vi "RunTest_NO.vi"(8 "error in (no error)":errorcluster, 11 "Prueba04 in":refnum<class "Prueba04.lvclass">) -> (0 "error out":errorcluster, 2 "resultado":string, 3 "Prueba04 out":refnum<class "Prueba04.lvclass">)   [LabVIEW 2019, in "Prueba04.lvclass"]
uses:
  Prueba04.lvclass
  Prueba/Prueba.lvclass
  Prueba/Queues/Private Controls/Estados.ctl
  Prueba/Queues/Private Controls/Control HMI Data Cluster.ctl
  Prueba/Queues/Private Controls/Queue FGV Action.ctl
  Prueba/Controles/FrecAmpGEN.ctl
  Control/Slide.ctl
panel:
  out "fila actual Z":i32
  out "frec_generar_Z2":string
  out "volt_generar_Z2":string
  out "frec_ref_Z_2":string="inicio"
  out "Vref_Z":dbl
  out "IndicadorAjuste_Z":dbl caption="Ajuste de amplitud [mV]"
  out "frecZ1":dbl
  out "cumple_no_cumple_Z":bool
  out "cumple_no_cumple_C":bool
  out "fila actual C":i32
  out "frec_generar_C2":string
  out "volt_generar_C2":string
  out "frec_ref_C":string="inicio"
  out "frecC1":dbl
  out "IndicadorAjuste_C":dbl caption="Ajuste de amplitud [mV]"
  out "Vref_C":dbl
  out "cumple_no_cumple_A":bool
  out "error out 2":errorcluster
  out "ponderacion_Z":bool
  out "ponderacion_C":bool
  out "volt_generar_A2":string
  out "FrecAmpGEN":T1
  out "Vref_A 2":dbl
  out "frecA1":dbl
  out "frec_generar_C2":string
  out "Voltajes_Ref_Z":string[](array[string])
  out "Voltajes_Ref_C":string[](array[string])
  out "fila actual Z":i32
  out "fila actual C":i32
  out "frec_ref_Z":string="inicio"
  out "frec_ref_C":string="inicio"
  out "frec_generar_A2":string
  out "fila actual A":i32
  out "Voltajes_Ref_A":string[](array[string])
  out "frec_ref_A":string="inicio"
  out "Vref_A":dbl
  out "IndicadorAjuste_A":dbl caption="Ajuste de amplitud [mV]"
  out "ponderacion_A":bool
  out "Tab":T2(tab)
  in  "go_A":bool
  in  "go_C":bool
  in  "go_Z":bool
  in  "seguir":bool
  out "no_cumple_prueba04":bool
  out "cumple_prueba04":bool
  out "estado_ensayo_A":string="Ensayo ya realizado"
  out "estado_ensayo_C":string="Ensayo ya realizado"
  out "estado_ensayo_Z":string="Ensayo ya realizado"
  in  "cb_frec_A_1":string(combo)="1000"
  in  "guardar_Vref_A":bool
  out "niveldBA_1":dbl=95.0
  out "rangoRefA_1":dbl=140.0
  in  "generarA1":bool
  in  "VoltAjuste_A":T3 caption="Ajuste de amplitud [mV]" scale=0.0..10.0
  out "voltMonA_1":dbl format="%#.1f"
  out "frecMonA_1":dbl format="%#.1f"
  in  "ir a resultados_A":bool
  in  "cb_frec_A_2":string(combo)="31,5"
  out "voltaje_A":dbl
  in  "generarA2":bool
  out "cumple_A":bool
  out "no_cumple_A":bool
  in  "ir a inicio desde A":bool
  in  "Tabla_A":string[][](table)
  out "voltMonA_2":dbl format="%#.1f"
  out "frecMonA_2":dbl format="%#.1f"
  in  "cb_frec_C_1":string(combo)="1000"
  in  "guardar_Vref_C":bool
  out "niveldBC_1":dbl
  out "rangoRefC_1":dbl
  in  "generarC1":bool
  in  "VoltAjuste_C":T3 caption="Ajuste de amplitud [mV]" scale=0.0..10.0
  out "voltMonC_1":dbl
  out "frecMonC_1":dbl
  in  "ir a resultados_C":bool
  in  "cb_frec_C_2":string(combo)="31,5"
  out "voltaje_C":dbl
  in  "generarC2":bool
  out "voltMonC_2":dbl
  out "frecMonC_2":dbl
  in  "Tabla_C":string[][](table)
  in  "ir a inicio desde C":bool
  out "cumple_C":bool
  out "no_cumple_C":bool
  in  "cb_frec_Z_1":string(combo)="1000"
  out "niveldBZ_1":dbl
  out "rangoRefZ_1":dbl
  in  "generarZ1":bool
  in  "VoltAjuste_Z":T3 caption="Ajuste de amplitud [mV]" scale=0.0..10.0
  out "voltMonZ_1":dbl
  out "frecMonZ_1":dbl
  in  "ir a resultados _Z":bool
  in  "guardar_Vref_Z":bool
  in  "cb_frec_Z_2":string(combo)="31,5"
  out "voltaje_Z":dbl
  in  "generarZ2":bool
  in  "ir a inicio desde Z":bool
  in  "Tabla_Z":string[][](table)
  out "voltMonZ_2":dbl
  out "frecMonZ_2":dbl
  out "cumple_Z":bool
  out "no_cumple_Z":bool
  # "Cumple"
  # "No Cumple"
  # "Ensayo Eléctrico Ponderación A"
  # "Ensayo Eléctrico Ponderación B"
  # "Ensayo Eléctrico Ponderación Z"
  # "Ensayo Eléctrico Ponderación A – Selección de Señal de referencia"
  # "Elección Señal de Referencia\nsegún marca y modelo de sonómetro"
  # "Nivel en dB"
  # "Rango Referencia"
  # "Frecuencia"
  # "Monitoreo"
  # "Frecuencia"
  # "Hz"
  # "Voltaje"
  # "V"
  # "Ensayo Eléctrico Ponderación A – Tabla de Resultados"
  # "Cumple"
  # "No Cumple"
  # "Hz"
  # "mV"
  # "Voltaje"
  # "Frecuencia"
  # "Ponderación A"
  # "Monitoreo"
  # "Frecuencia"
  # "Hz"
  # "Voltaje"
  # "V"
  # "Ensayo Eléctrico Ponderación C – Selección de Señal de referencia"
  # "Elección Señal de Referencia\nsegún marca y modelo de sonómetro"
  # "Nivel en dB"
  # "Rango Referencia"
  # "Frecuencia"
  # "Monitoreo"
  # "Frecuencia"
  # "Hz"
  # "Voltaje"
  # "V"
  # "Ensayo Eléctrico Ponderación C – Tabla de Resultados"
  # "Cumple"
  # "No Cumple"
  # "Hz"
  # "mV"
  # "Voltaje"
  # "Frecuencia"
  # "Monitoreo"
  # "Frecuencia"
  # "Hz"
  # "Voltaje"
  # "V"
  # "Ponderación C"
  # "Ensayo Eléctrico Ponderación Z – Selección de Señal de referencia"
  # "Elección Señal de Referencia\nsegún marca y modelo de sonómetro"
  # "Nivel en dB"
  # "Rango Referencia"
  # "Frecuencia"
  # "Monitoreo"
  # "Frecuencia"
  # "Hz"
  # "Voltaje"
  # "V"
  # "Ensayo Eléctrico Ponderación Z – Tabla de Resultados"
  # "Cumple"
  # "No Cumple"
  # "Hz"
  # "mV"
  # "Voltaje"
  # "Frecuencia"
  # "Ponderación Z"
  # "Monitoreo"
  # "Frecuencia"
  # "Hz"
  # "Voltaje"
  # "V"
  # "4. Ensayo  de las ponderaciones frecuenciales con señales eléctricas. IEC 61672-3: 2006 Cláusula 12"
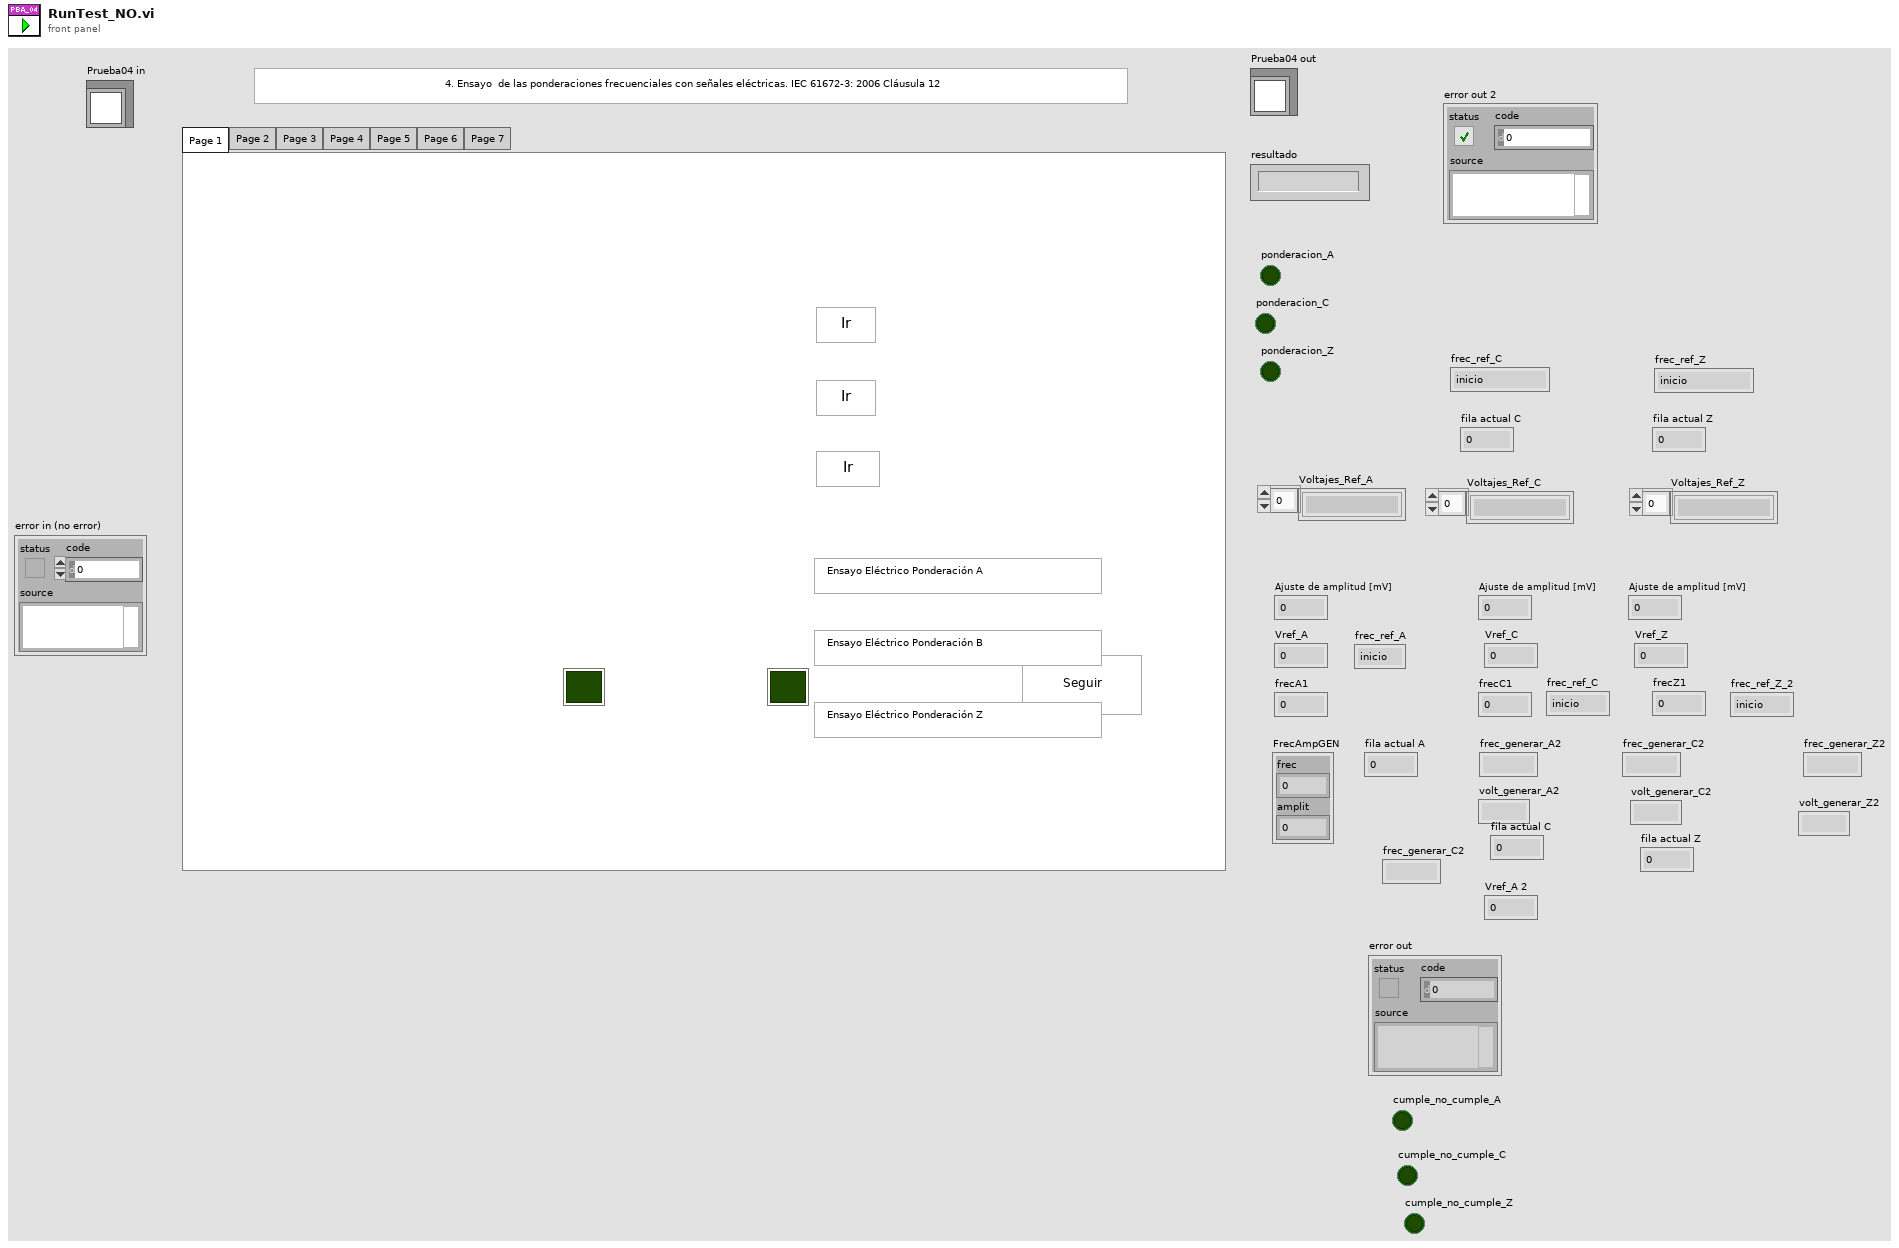
[diagram p1: front panel]
types:
  T1 = typedef "Prueba04.lvclass/FrecAmpGEN.ctl" = cluster{"frec":dbl, "amplit":dbl}
  T2 = enum32{"Page 1", "Page 2", "Page 3", "Page 4", "Page 5", "Page 6", "Page 7"}
  T3 = typedef "Prueba04.lvclass/Slide.ctl" = dbl
  T4 = cluster{"Medido":dbl, "Ref":dbl, "Incert_exp":dbl, "Tol+":dbl, "Tol-":dbl, "fila":i32}
  T5 = typedef "Queue FGV Action.ctl" = enum16{"Set", "Get", "Release"}
  T6 = enum8{"Enabled", "Disabled", "Disabled and Grayed Out"}
  T7 = typedef "Control HMI Data Cluster.ctl" = cluster{"Estados":T8, "Data":variant}
  T8 = typedef "Estados.ctl" = enum16{"CargaReferencias", "LeerArchivoConfiguracion", "RevisaTipoGenerador", "inicio", "conf_instru", "escribe_frec", "lee_BD", "lee_referencia", "guardarVrefA", "guardarVrefC", "guardarVrefZ", "FrecAmp_A1", "FrecAmp_C1", "FrecAmp_Z1", "FrecAmp_A2", "FrecAmp_C2", "FrecAmp_Z2", "iniciarGEN", "monitoreo", "detenerGEN", "crea_voltajes_prueba_A", "crea_voltajes_prueba_C", "crea_voltajes_prueba_Z", "voltajeInicialA2", "voltajeInicialC2", "voltajeInicialZ2", "actualizarVrefA", "actualizarVrefC", "actualizarVrefZ", "ingresaMedicionesA", "ingresaMedicionesC", "ingresaMedicionesZ", "cumplimiento", "listo_evaluar", "evaluar", "final", "guardaMedicionesA", "guardaMedicionesC", "guardaMedicionesZ", "ultimaFrec", "generaA2", "detieneA2", "salir", "Error"}
  T9 = cluster{"Medido":dbl, "Error":dbl, "Ref":dbl, "Incert_exp":dbl, "Tol+":dbl, "Tol-":dbl, "fila":i32}
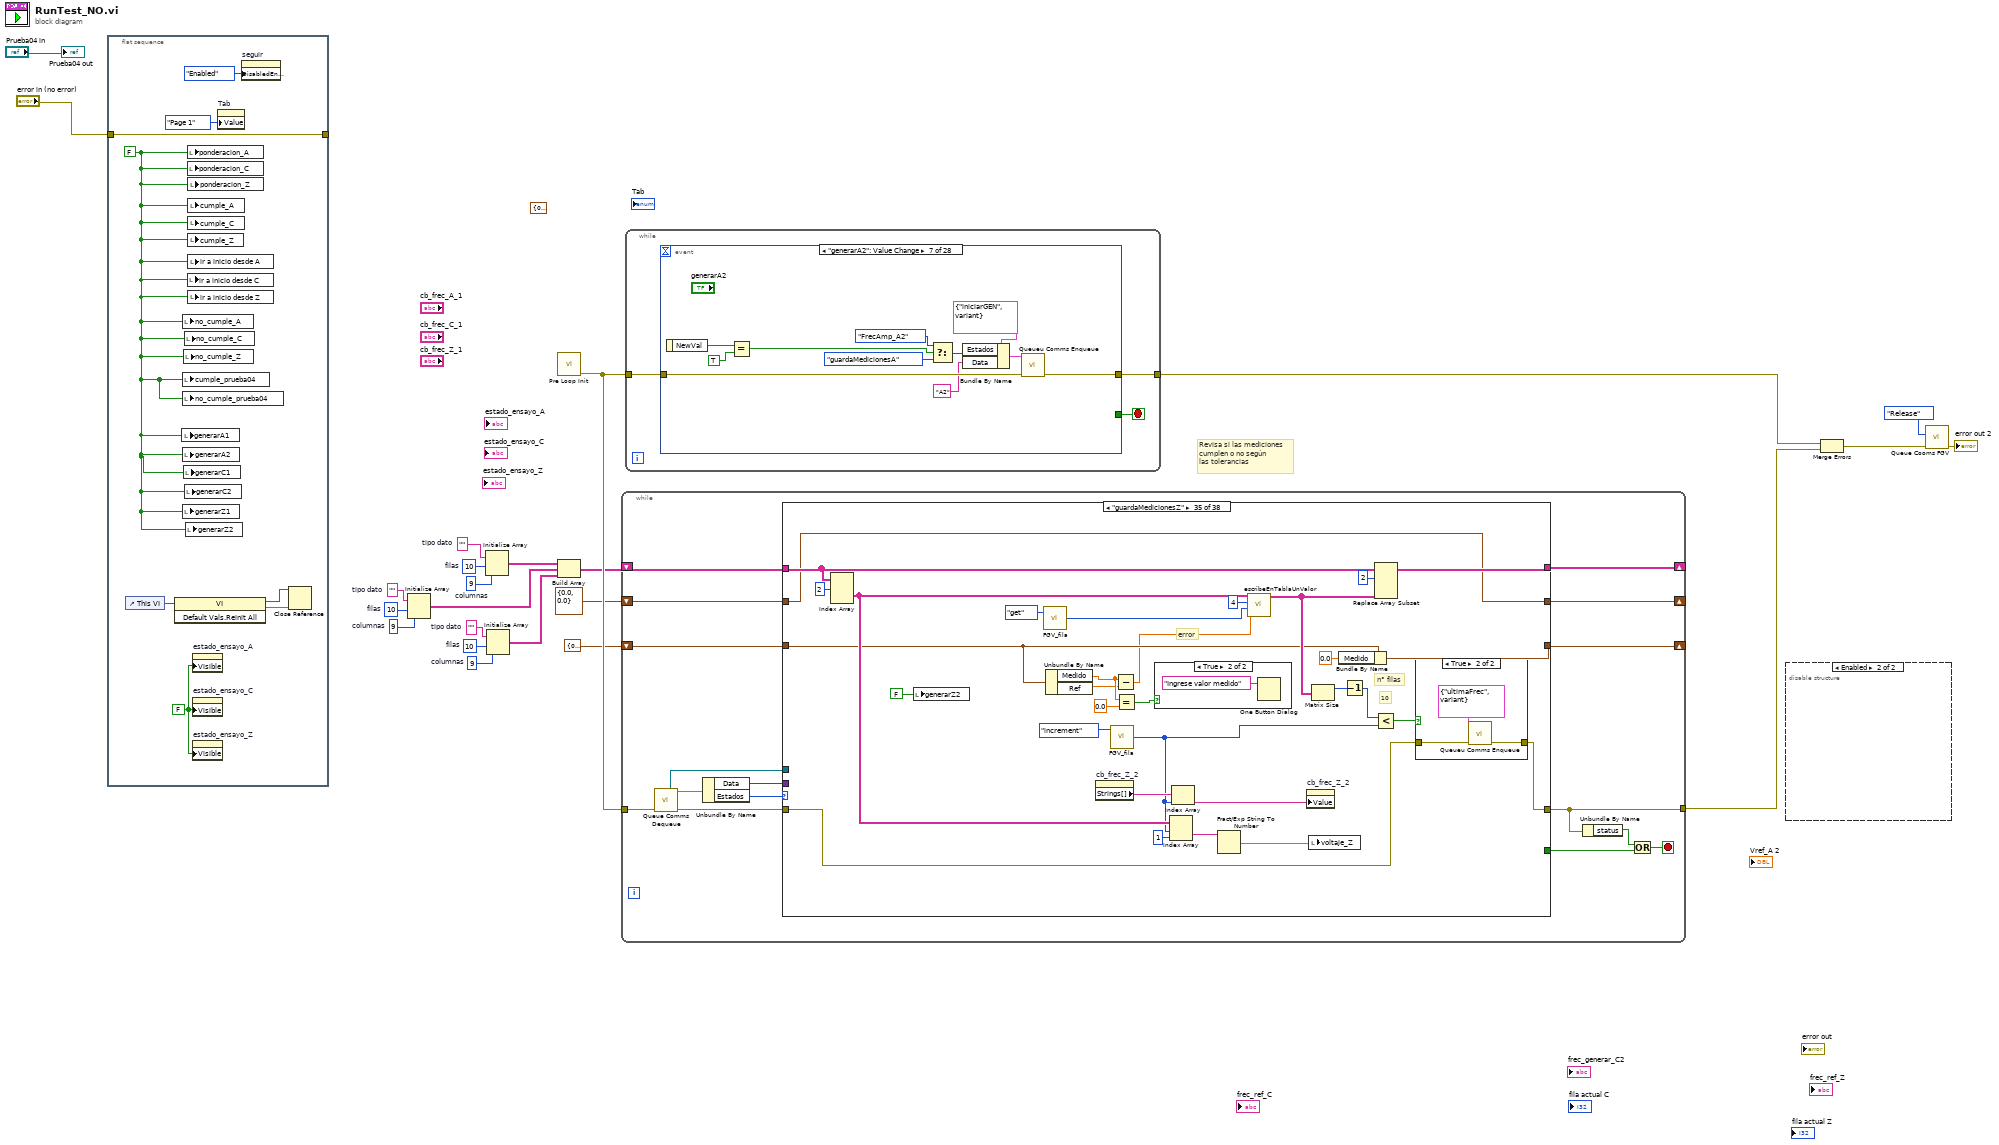
[diagram p0: block diagram]
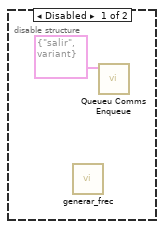
[diagram p2: hidden frame]
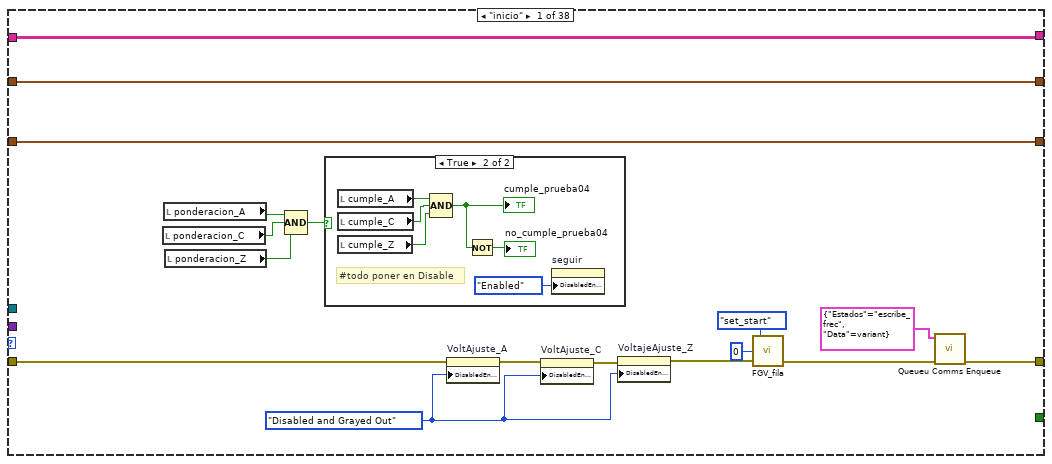
[diagram p3: hidden frame]
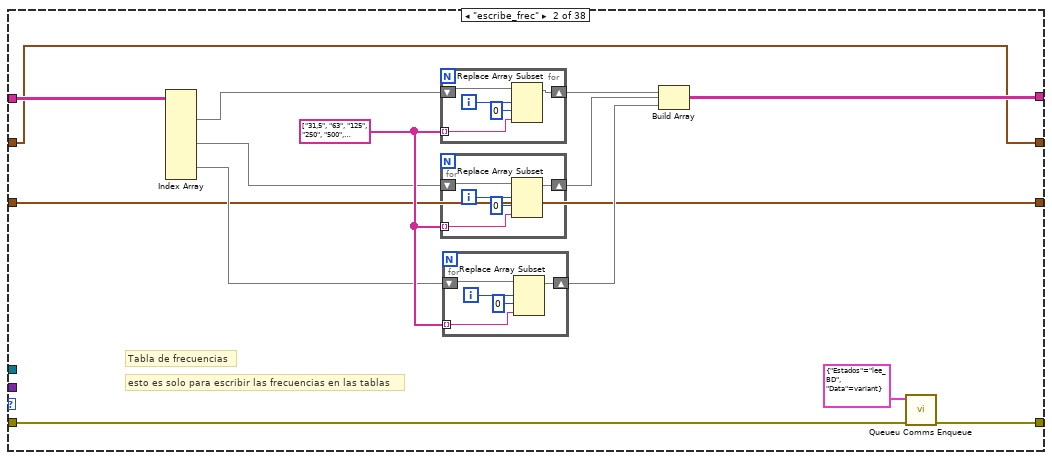
[diagram p5: hidden frame]
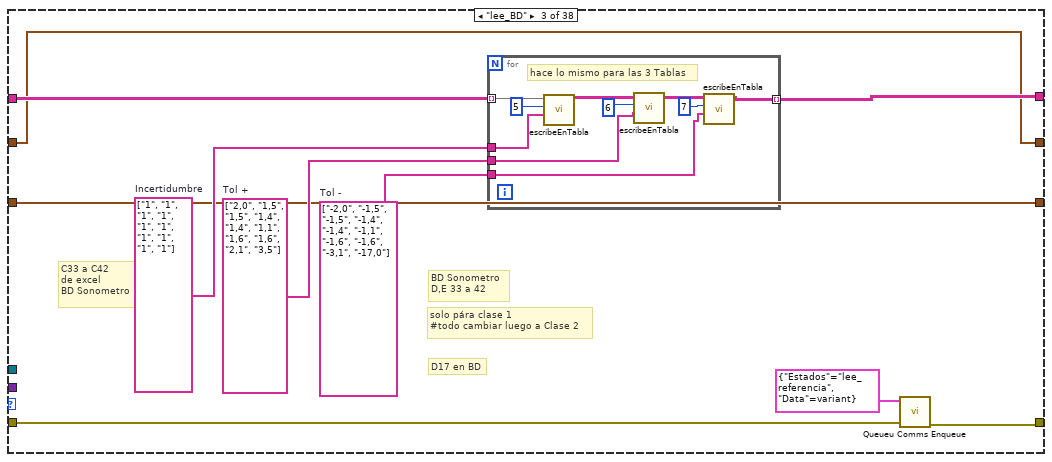
[diagram p6: hidden frame]
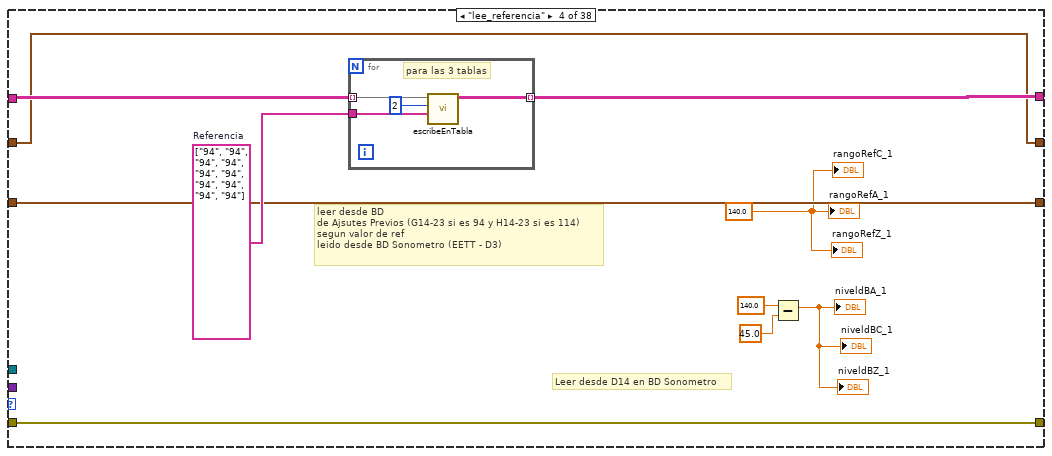
[diagram p7: hidden frame]
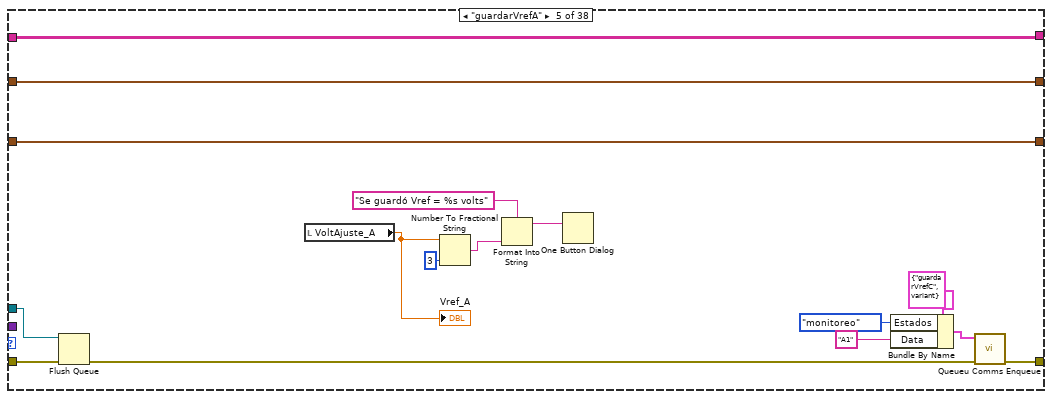
[diagram p8: hidden frame]
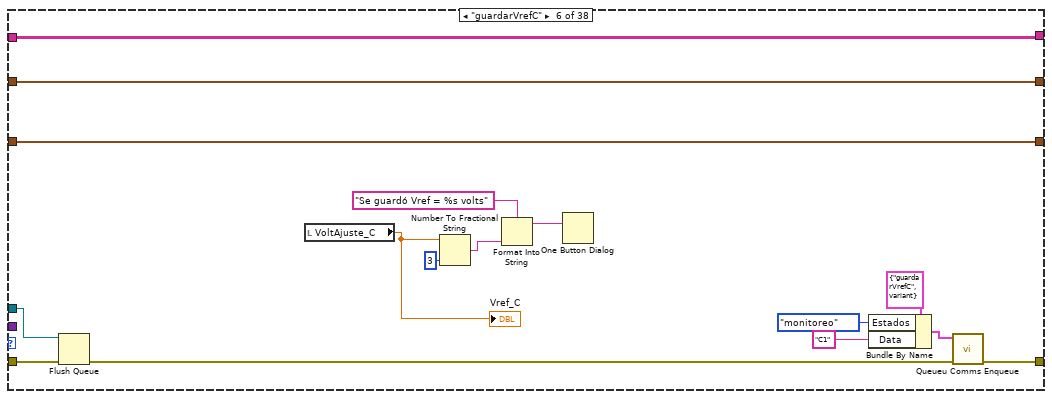
[diagram p9: hidden frame]
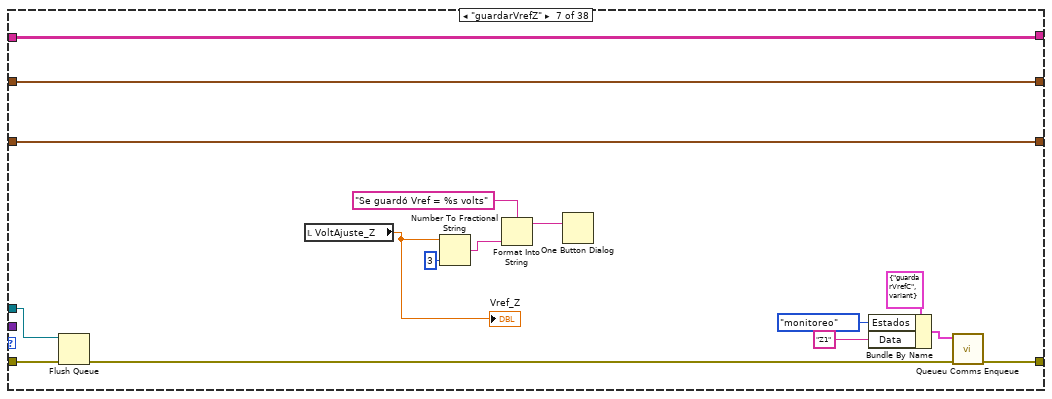
[diagram p10: hidden frame]
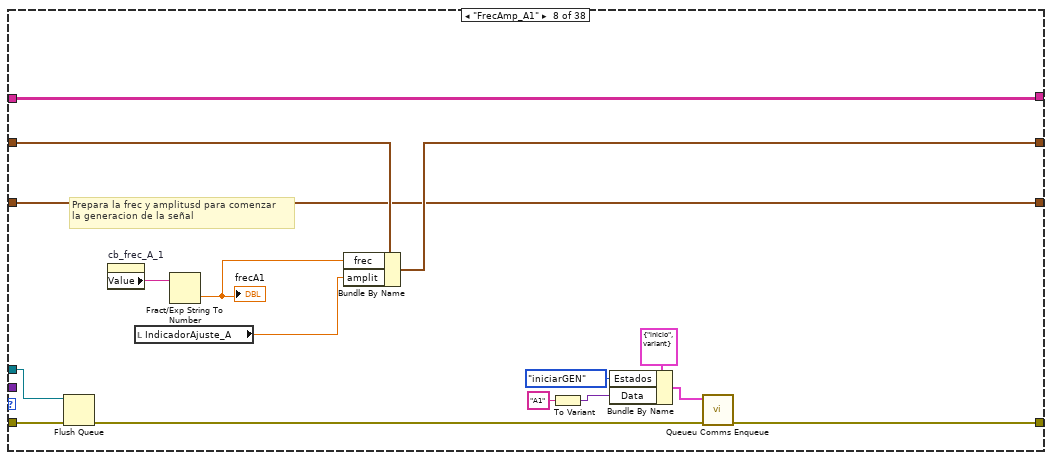
[diagram p11: hidden frame]
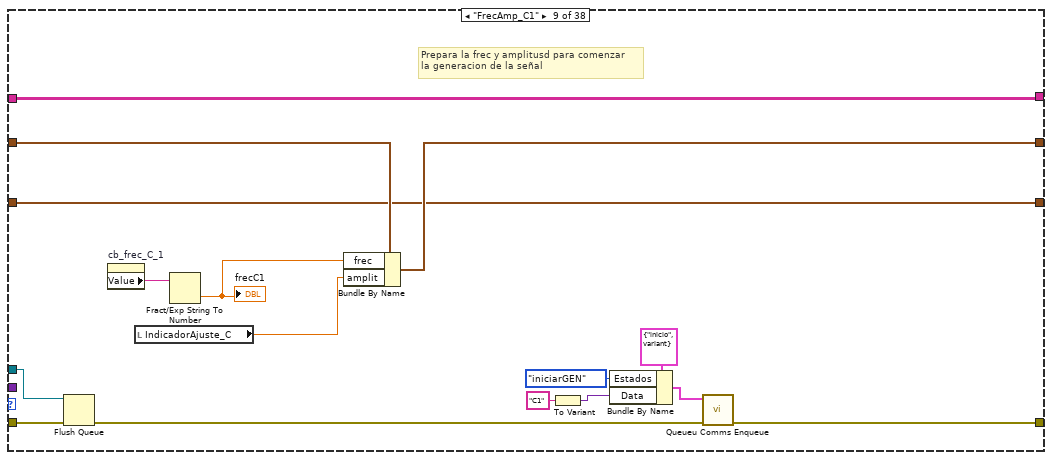
[diagram p12: hidden frame]
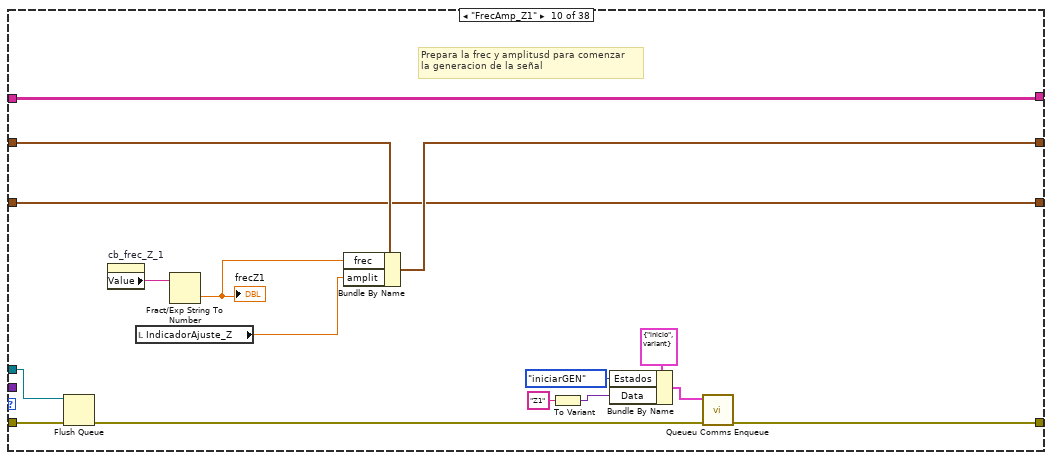
[diagram p13: hidden frame]
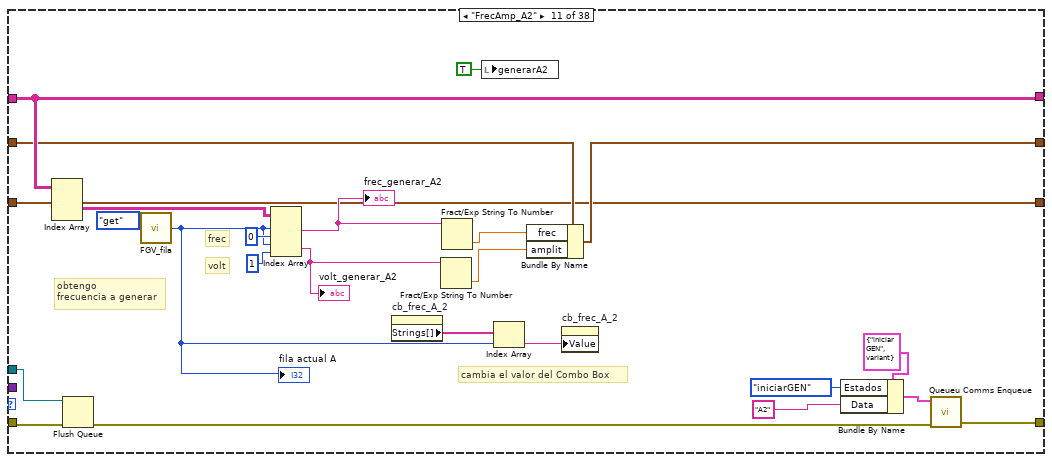
[diagram p14: hidden frame]
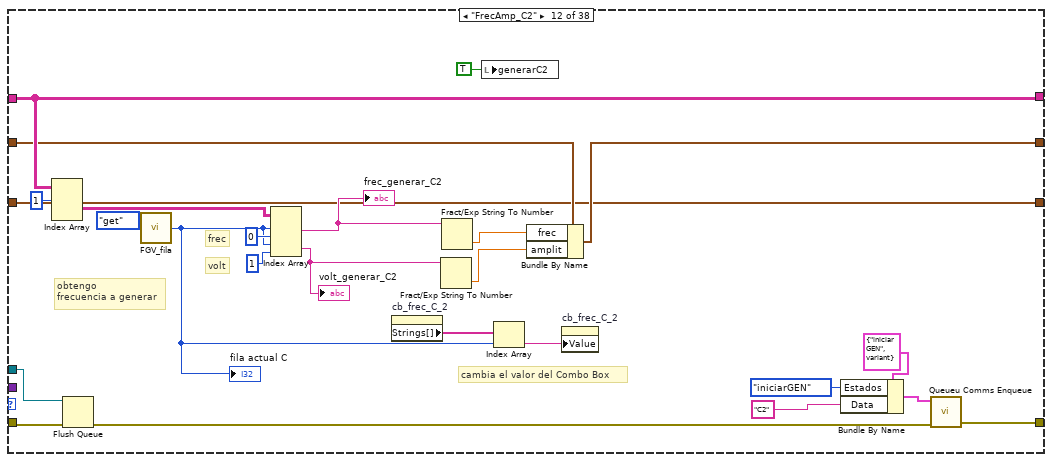
[diagram p15: hidden frame]
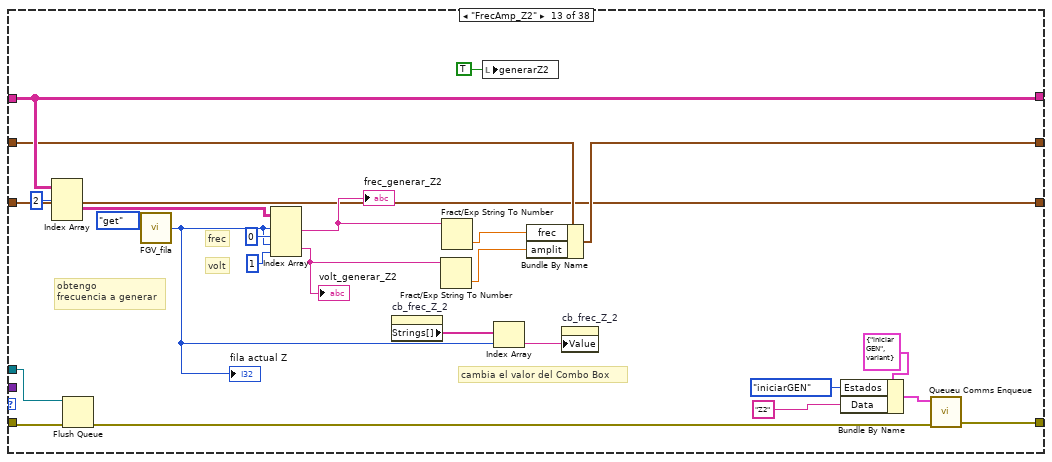
[diagram p16: hidden frame]
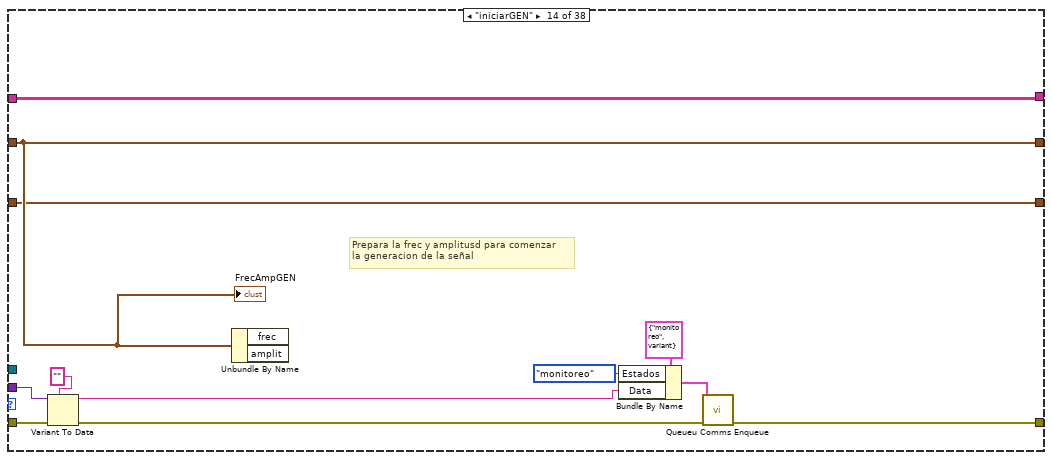
[diagram p17: hidden frame]
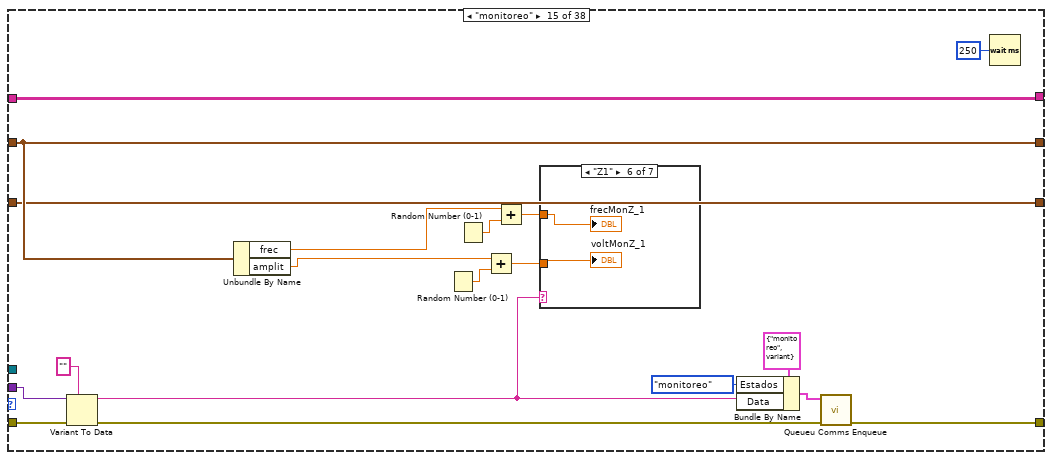
[diagram p18: hidden frame]
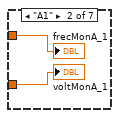
[diagram p20: hidden frame]
diagram:
  w12 = 9  # columnas
  w13 = 10  # filas
  w11 = ""  # tipo dato
  w9 = 9  # columnas
  w8 = 10  # filas
  w10 = ""  # tipo dato
  w6 = 9  # columnas
  w7 = 10  # filas
  w5 = ""  # tipo dato
  (unwired) T4 {"Medido"=0.0, "Ref"=0.0, "Incert_exp"=0.0, "Tol+"=0.0, "Tol-"=0.0, "fila"=0}
  # "Revisa si las mediciones\ncumplen o no según\nlas tolerancias"
  n1 = flat-sequence {
    tunnel: "error in (no error)" -> [w30]
    tunnel: [w30] -> _
    frame #0 {
      w24 = FALSE ("Visible")
      w25 = FALSE ("cumple_A")
      n2 = control-ref of="This VI"() -> (w27:refnum<vi>)
      n3 = invoke class="VI" method="Default Vals.Reinit All"(reference=w27) -> (reference out=w26:refnum<vi>, error out=w28:errorcluster)  [unwired: 2 in, 1 out]
      n4 = local write "generarA1"(w25) -> ()
      n5 = local write "no_cumple_A"(w25) -> ()
      n6 = local write "cumple_prueba04"(w25) -> ()
      n7 = local write "no_cumple_prueba04"(w25) -> ()
      n8 = local write "generarA2"(w25) -> ()
      n9 = local write "generarZ1"(w25) -> ()
      n10 = local write "no_cumple_Z"(w25) -> ()
      n11 = local write "generarC1"(w25) -> ()
      n12 = local write "no_cumple_C"(w25) -> ()
      n13 = local write "generarC2"(w25) -> ()
      n14 = local write "generarZ2"(w25) -> ()
      n15 = local write "ponderacion_A"(w25) -> ()
      n16 = local write "ponderacion_C"(w25) -> ()
      n17 = local write "ir a inicio desde C"(w25) -> ()
      n18 = local write "ponderacion_Z"(w25) -> ()
      n19 = local write "cumple_A"(w25) -> ()
      n20 = local write "cumple_C"(w25) -> ()
      n21 = local write "cumple_Z"(w25) -> ()
      n22 = local write "ir a inicio desde A"(w25) -> ()
      n23 = local write "ir a inicio desde Z"(w25) -> ()
      n24 = property on="estado_ensayo_A" class="Str"("Visible"=w24) -> ()  [unwired: 2 in, 2 out]
      n25 = property on="estado_ensayo_C" class="Str"("Visible"=w24) -> ()  [unwired: 2 in, 2 out]
      n26 = property on="estado_ensayo_Z" class="Str"("Visible"=w24) -> ()  [unwired: 2 in, 2 out]
      n27 = property on="Tab" class="TabCtl (strict)"("Value"=T2."Page 1" ("Tab_Prueba04")) -> ()  [unwired: 2 in, 2 out]
      n28 = property on="seguir" class="Bool"("DisabledEnum"=T6."Enabled" ("Disabled")) -> ()  [unwired: 2 in, 2 out]
      n29 = Close Reference(reference=w26, error in (no error)=w28) -> ()  [unwired: 1 out]
    }
  }
  n30 = Initialize Array(w10, w8, w9) -> (w15:string[][])
  n31 = Initialize Array(w5, w7, w6) -> (w14:string[][])
  n32 = Initialize Array(w11, w13, w12) -> (w16:string[][])
  n33 = call "Pre Loop Init.vi"() -> ("error out"=w21:errorcluster)  [unwired: 11 in]
  n34 = Build Array(w14, w15, w16) -> (w4:string[][][])
  n35 = while {
    tunnel: w21 -> [w45]
    tunnel: [w43] -> w19
    shift-right: [w38] -> _
    shift-left: w4 -> [w39]
    shift-right: [w36] -> _
    shift-left: T1 {"frec"=0.0, "amplit"=0.0} ("ParamGeneracion") -> [w37]
    shift-right: [w32] -> _
    shift-left: T4 {"Medido"=0.0, "Ref"=0.0, "Incert_exp"=0.0, "Tol+"=0.0, "Tol-"=0.0, "fila"=0} -> [w33]
    stop <- w40 stop-if-true
    n36 = call "Queue Comms Dequeue.vi"("error in"=w45) -> ("error out"=w44:errorcluster, "Data Out"=w35:T7, "queue out"=w34:refnum<queue>)  [unwired: 8 in]
    n37 = Unbundle By Name(w35) -> ("Data"=w46:variant, "Estados"=w47:T8)
    n38 = case shown="\"guardaMedicionesZ\"" w47 {
      tunnel: w46 -> [_ _ _ _ _ _ _ _ _ _ _ _ _ w306 w324 _ _ _ _ _ _ _ _ _ _ w515 w538 w561 w578 w594 w656 _ _ _ _ _ _ _]
      tunnel: [_ _ _ _ _ _ _ _ _ _ _ _ _ _ _ _ _ _ _ _ _ _ _ _ _ _ _ _ _ _ _ _ _ _ _ _ TRUE _] -> w41
      tunnel: [w60 w74 w103 w124 w135 w155 w171 w194 w210 w226 w235 w260 w285 w313 w317 w349 w360 w387 w413 w435 w445 w451 w465 w476 w487 w510 w533 w556 w568 w596 w660 w704 w711 w749 w787 w824 w832 w837] -> w43
      tunnel: w44 -> [w49 w73 w102 w124 w144 w160 w176 w195 w211 w227 w233 w258 w283 w314 w333 w353 w361 w388 w414 w435 w445 w452 w466 w477 w488 w496 w519 w542 w579 w600 w664 w704 w712 w750 w788 w820 w832 w837]
      tunnel: w39 -> [w58 w77 w106 w126 w149 w165 w181 w197 w213 w229 w249 w274 w299 w315 w334 w354 w367 w393 w419 w441 w450 w460 w471 w482 w493 w513 w536 w559 w576 w597 w661 w703 w730 w768 w806 w828 w831 w836]
      tunnel: [w58 w76 w105 w125 w149 w165 w181 w197 w213 w229 w249 w274 w299 w315 w334 w354 w366 w392 w418 w441 w450 w460 w471 w482 w493 w512 w535 w558 w572 w597 w661 w703 w729 w767 w805 w828 w831 w836] -> w38
      tunnel: w37 -> [w57 w72 w101 w123 w143 w159 w175 w193 w209 w225 w244 w269 w294 w312 w325 w352 w359 w386 w412 w434 w444 w455 w470 w481 w492 w516 w539 w562 w581 w599 w663 w702 w720 w758 w796 w827 w830 w835]
      tunnel: [w57 w72 w101 w123 w143 w159 w175 w191 w207 w223 w239 w264 w289 w312 w325 w352 w359 w386 w412 w434 w444 w455 w470 w481 w492 w516 w539 w562 w581 w599 w663 w702 w720 w758 w796 w827 w830 w835] -> w36
      tunnel: w34 -> [_ _ _ _ w141 w158 w174 w183 w199 w215 w231 w256 w281 _ _ w348 w357 w384 w410 _ _ _ _ _ _ w494 w517 w540 _ _ _ _ _ _ _ _ _ _]
      tunnel: w33 -> [w55 w71 w100 w122 w140 w157 w173 w182 w198 w214 w230 w255 w280 w304 w316 w347 w356 w383 w409 w433 w443 w454 w469 w480 w491 w501 w524 w547 w574 w598 w662 w701 w709 w747 w785 w821 w829 w834]
      tunnel: [w55 w71 w100 w122 w140 w157 w173 w182 w198 w214 w230 w255 w280 w304 w316 w347 w356 w383 w409 w433 w443 w454 w469 w480 w491 w497 w520 w543 w573 w598 w662 w701 w707 w745 w783 w821 w829 w834] -> w32
      frame "inicio" {
        w50 = T6."Disabled and Grayed Out" ("Disabled")
        n39 = local read "ponderacion_C"() -> (w56:bool)
        n40 = local read "ponderacion_A"() -> (w63:bool)
        n41 = local read "ponderacion_Z"() -> (w64:bool)
        n42 = Compound Arithmetic op=AND(w63, w56, w64) -> (w48:bool)
        n43 = case shown="True" w48 {
          frame False {
          }
          frame True {
            # "#todo poner en Disable"
            n44 = local read "cumple_A"() -> (w70:bool)
            n45 = local read "cumple_C"() -> (w66:bool)
            n46 = local read "cumple_Z"() -> (w65:bool)
            n47 = Compound Arithmetic op=AND(w70, w66, w65) -> (w67:bool)
            "cumple_prueba04" <- w67
            n48 = Not(x=w67) -> (.not. x?=→"no_cumple_prueba04":bool)
            n49 = property on="seguir" class="Bool"("DisabledEnum"=T6."Enabled" ("Disabled")) -> ()  [unwired: 2 in, 2 out]
          }
        }
        n50 = property on="VoltAjuste_A" class="Slide (strict)"(error in=w49, "DisabledEnum"=w50) -> (error out=w53:errorcluster)  [unwired: 1 in, 1 out]
        n51 = property on="VoltAjuste_C" class="Slide (strict)"(error in=w53, "DisabledEnum"=w50) -> (error out=w52:errorcluster)  [unwired: 1 in, 1 out]
        n52 = property on="VoltajeAjuste_Z" class="Slide (strict)"(error in=w52, "DisabledEnum"=w50) -> (error out=w51:errorcluster)  [unwired: 1 in, 1 out]
        n53 = call "FGV_fila.vi"("error in (no error)"=w51, "fila_inicial"=0, "action"=enum16{"increment", "set_start", "get"}."set_start") -> ("error out"=w54:errorcluster)  [unwired: 1 in, 1 out]
        n54 = call "Queueu Comms Enqueue.vi"("error in"=w54, "Element"=T7 {"Estados"=enum."escribe_frec", "Data"=variant} ("Module Dat Cluster")) -> ("error out"=w60:errorcluster)  [unwired: 8 in, 1 out]
      }
      frame "escribe_frec" {
        w84 = string[] ["31,5", "63", "125", "250", "500", "1000", "2000", "4000", "8000", "16000"]
        # "esto es solo para escribir las frecuencias en las tablas"
        # "Tabla de frecuencias"
        n55 = Index Array(array=w77) -> (element #1=w78:string[][], element #2=w79:string[][], element #3=w80:string[][])  [unwired: 9 in]
        n56 = for {
          shift-right: [w98] -> w81
          shift-left: w78 -> [w99]
          tunnel: w84 -> [w95] mode=indexing
          i -> [w97]
          n57 = Replace Array Subset(array=w99, new element=w95, index (row)=w97, index (col)=0 ("disabled index (col)")) -> (w98:string[][])
        }
        n58 = for {
          shift-right: [w93] -> w82
          shift-left: w79 -> [w94]
          tunnel: w84 -> [w90] mode=indexing
          i -> [w92]
          n59 = Replace Array Subset(array=w94, new element=w90, index (row)=w92, index (col)=0 ("disabled index (col)")) -> (w93:string[][])
        }
        n60 = for {
          shift-right: [w88] -> w83
          shift-left: w80 -> [w89]
          tunnel: w84 -> [w85] mode=indexing
          i -> [w87]
          n61 = Replace Array Subset(array=w89, new element=w85, index (row)=w87, index (col)=0 ("disabled index (col)")) -> (w88:string[][])
        }
        n62 = Build Array(w81, w82, w83) -> (w76:string[][][])
        n63 = call "Queueu Comms Enqueue.vi"("error in"=w73, "Element"=T7 {"Estados"=enum."lee_BD", "Data"=variant} ("Module Dat Cluster")) -> ("error out"=w74:errorcluster)  [unwired: 8 in, 1 out]
      }
      frame "lee_BD" {
        w109 = string[] ["-2,0", "-1,5", "-1,5", "-1,4", "-1,4", "-1,1", "-1,6", "-1,6", "-3,1", "-17,0"]  # Tol -
        w108 = string[] ["2,0", "1,5", "1,5", "1,4", "1,4", "1,1", "1,6", "1,6", "2,1", "3,5"]  # Tol +
        w107 = string[] ["1", "1", "1", "1", "1", "1", "1", "1", "1", "1"]  # Incertidumbre
        # "D17 en BD"
        # "BD Sonometro\nD,E 33 a 42"
        # "solo pára clase 1\n#todo cambiar luego a Clase 2"
        # "C33 a C42\nde excel\nBD Sonometro"
        n64 = for {
          tunnel: w106 -> [w118] mode=indexing
          tunnel: w107 -> [w116]
          tunnel: w108 -> [w113]
          tunnel: w109 -> [w110]
          tunnel: [w111] -> w105 mode=indexing
          # "hace lo mismo para las 3 Tablas"
          n65 = call "escribeEnTabla.vi"("parametros"=w116, "col"=5, "tabla in"=w118) -> ("tabla out"=w115:string[][])  [unwired: 8 in]
          n66 = call "escribeEnTabla.vi"("parametros"=w113, "col"=6, "tabla in"=w115) -> ("tabla out"=w112:string[][])  [unwired: 8 in]
          n67 = call "escribeEnTabla.vi"("parametros"=w110, "col"=7, "tabla in"=w112) -> ("tabla out"=w111:string[][])  [unwired: 8 in]
        }
        n68 = call "Queueu Comms Enqueue.vi"("error in"=w102, "Element"=T7 {"Estados"=enum."lee_referencia", "Data"=variant} ("Module Dat Cluster")) -> ("error out"=w103:errorcluster)  [unwired: 8 in, 1 out]
      }
      frame "lee_referencia" {
        w121 = 140.0 ("rangoRefA_1")
        w127 = string[] ["94", "94", "94", "94", "94", "94", "94", "94", "94", "94"]  # Referencia
        # "Leer desde D14 en BD Sonometro"
        # "leer desde BD\nde Ajsutes Previos (G14-23 si es 94 y H14-23 si es 114)  \nsegun valor de ref\nleido desde BD Sonometro (EETT - D3)"
        n69 = for {
          tunnel: w126 -> [w133] mode=indexing
          tunnel: [w132] -> w125 mode=indexing
          tunnel: w127 -> [w130]
          # "para las 3 tablas"
          n70 = call "escribeEnTabla.vi"("parametros"=w130, "col"=2, "tabla in"=w133) -> ("tabla out"=w132:string[][])  [unwired: 8 in]
        }
        n71 = Subtract(x=140.0 ("rangoRefA_1"), y=45.0) -> (x-y=→"niveldBA_1" →"niveldBC_1" →"niveldBZ_1":dbl)
        "rangoRefA_1" <- w121
        "rangoRefC_1" <- w121
        "rangoRefZ_1" <- w121
      }
      frame "guardarVrefA" {
        n72 = Flush Queue(queue=w141, error in (no error)=w144) -> (error out=w134:errorcluster)  [unwired: 2 out]
        n73 = local read "VoltAjuste_A"() -> (w142:T3)
        "Vref_A" <- w142
        n74 = Number To Fractional String(number=w142, precision (6)=i16 3) -> (F-format string=w148:string)  [unwired: 2 in]
        n75 = Format Into String(format string="Se guardó Vref = %s volts", w148) -> (resulting string=w145:string)  [unwired: 2 in, 1 out]
        n76 = One Button Dialog(message=w145) -> ()  [unwired: 1 in, 1 out]
        n77 = Bundle By Name(cluster=T7 {"Estados"=enum."guardarVrefC", "Data"=variant} ("Module Dat Cluster"), "Estados"=Estados."monitoreo", "Data"="A1" ("format string")) -> (w139:T7)
        n78 = call "Queueu Comms Enqueue.vi"("error in"=w134, "Element"=w139) -> ("error out"=w135:errorcluster)  [unwired: 8 in, 1 out]
      }
      frame "guardarVrefC" {
        n79 = Flush Queue(queue=w158, error in (no error)=w160) -> (error out=w154:errorcluster)  [unwired: 2 out]
        n80 = local read "VoltAjuste_C"() -> (w156:T3)
        "Vref_C" <- w156
        n81 = Number To Fractional String(number=w156, precision (6)=i16 3) -> (F-format string=w164:string)  [unwired: 2 in]
        n82 = Format Into String(format string="Se guardó Vref = %s volts", w164) -> (resulting string=w161:string)  [unwired: 2 in, 1 out]
        n83 = One Button Dialog(message=w161) -> ()  [unwired: 1 in, 1 out]
        n84 = Bundle By Name(cluster=T7 {"Estados"=enum."guardarVrefC", "Data"=variant} ("Module Dat Cluster"), "Estados"=Estados."monitoreo", "Data"="C1" ("format string")) -> (w152:T7)
        n85 = call "Queueu Comms Enqueue.vi"("error in"=w154, "Element"=w152) -> ("error out"=w155:errorcluster)  [unwired: 8 in, 1 out]
      }
      frame "guardarVrefZ" {
        n86 = Flush Queue(queue=w174, error in (no error)=w176) -> (error out=w170:errorcluster)  [unwired: 2 out]
        n87 = local read "VoltAjuste_Z"() -> (w172:T3)
        "Vref_Z" <- w172
        n88 = Number To Fractional String(number=w172, precision (6)=i16 3) -> (F-format string=w180:string)  [unwired: 2 in]
        n89 = Format Into String(format string="Se guardó Vref = %s volts", w180) -> (resulting string=w177:string)  [unwired: 2 in, 1 out]
        n90 = One Button Dialog(message=w177) -> ()  [unwired: 1 in, 1 out]
        n91 = Bundle By Name(cluster=T7 {"Estados"=enum."guardarVrefC", "Data"=variant} ("Module Dat Cluster"), "Estados"=Estados."monitoreo", "Data"="Z1" ("format string")) -> (w168:T7)
        n92 = call "Queueu Comms Enqueue.vi"("error in"=w170, "Element"=w168) -> ("error out"=w171:errorcluster)  [unwired: 8 in, 1 out]
      }
      frame "FrecAmp_A1" {
        # "Prepara la frec y amplitusd para comenzar\nla generacion de la señal"
        n93 = Flush Queue(queue=w183, error in (no error)=w195) -> (error out=w184:errorcluster)  [unwired: 2 out]
        n94 = property on="cb_frec_A_1" class="CmbBox"() -> ("Value"=w196:string)  [unwired: 2 in, 2 out]
        n95 = local read "IndicadorAjuste_A"() -> (w185:dbl)
        n96 = Fract/Exp String To Number(string=w196) -> (number=w192:dbl)  [unwired: 3 in, 1 out]
        "frecA1" <- w192
        n97 = Bundle By Name(cluster=w193, "frec"=w192, "amplit"=w185) -> (w191:T1)
        n98 = To Variant(anything="A1" ("message")) -> (Variant=w186:variant)
        n99 = Bundle By Name(cluster=T7 {"Estados"=enum."inicio", "Data"=variant} ("Element"), "Estados"=Estados."iniciarGEN", "Data"=w186) -> (w188:T7)
        n100 = call "Queueu Comms Enqueue.vi"("error in"=w184, "Element"=w188) -> ("error out"=w194:errorcluster)  [unwired: 8 in, 1 out]
      }
      frame "FrecAmp_C1" {
        # "Prepara la frec y amplitusd para comenzar\nla generacion de la señal"
        n101 = Flush Queue(queue=w199, error in (no error)=w211) -> (error out=w200:errorcluster)  [unwired: 2 out]
        n102 = property on="cb_frec_C_1" class="CmbBox"() -> ("Value"=w212:string)  [unwired: 2 in, 2 out]
        n103 = local read "IndicadorAjuste_C"() -> (w201:dbl)
        n104 = Fract/Exp String To Number(string=w212) -> (number=w208:dbl)  [unwired: 3 in, 1 out]
        "frecC1" <- w208
        n105 = Bundle By Name(cluster=w209, "frec"=w208, "amplit"=w201) -> (w207:T1)
        n106 = To Variant(anything="C1" ("message")) -> (Variant=w202:variant)
        n107 = Bundle By Name(cluster=T7 {"Estados"=enum."inicio", "Data"=variant} ("Element"), "Estados"=Estados."iniciarGEN", "Data"=w202) -> (w204:T7)
        n108 = call "Queueu Comms Enqueue.vi"("error in"=w200, "Element"=w204) -> ("error out"=w210:errorcluster)  [unwired: 8 in, 1 out]
      }
      frame "FrecAmp_Z1" {
        # "Prepara la frec y amplitusd para comenzar\nla generacion de la señal"
        n109 = Flush Queue(queue=w215, error in (no error)=w227) -> (error out=w216:errorcluster)  [unwired: 2 out]
        n110 = property on="cb_frec_Z_1" class="CmbBox"() -> ("Value"=w228:string)  [unwired: 2 in, 2 out]
        n111 = local read "IndicadorAjuste_Z"() -> (w217:dbl)
        n112 = Fract/Exp String To Number(string=w228) -> (number=w224:dbl)  [unwired: 3 in, 1 out]
        "frecZ1" <- w224
        n113 = Bundle By Name(cluster=w225, "frec"=w224, "amplit"=w217) -> (w223:T1)
        n114 = To Variant(anything="Z1" ("message")) -> (Variant=w218:variant)
        n115 = Bundle By Name(cluster=T7 {"Estados"=enum."inicio", "Data"=variant} ("Element"), "Estados"=Estados."iniciarGEN", "Data"=w218) -> (w220:T7)
        n116 = call "Queueu Comms Enqueue.vi"("error in"=w216, "Element"=w220) -> ("error out"=w226:errorcluster)  [unwired: 8 in, 1 out]
      }
      frame "FrecAmp_A2" {
        # "volt"
        # "frec"
        # "cambia el valor del Combo Box"
        # "obtengo \nfrecuencia a generar"
        n117 = Index Array(array=w249) -> (element=w248:string[][])  [unwired: 3 in]
        n118 = Flush Queue(queue=w231, error in (no error)=w233) -> (error out=w232:errorcluster)  [unwired: 2 out]
        n119 = call "FGV_fila.vi"("action"=enum16{"increment", "set_start", "get"}."get") -> ("fila out"=w246:i32)  [unwired: 3 in, 1 out]
        "fila actual A" <- w246
        n120 = Index Array(array=w248, index (row) #1=w246, index (col) #1=0 ("disabled index (col)"), index (row) #2=w246, index (col) #2=1 ("disabled index (col)")) -> (element #1=w243:string, element #2=w242:string)
        "frec_generar_A2" <- w243
        "volt_generar_A2" <- w242
        n121 = property on="cb_frec_A_2" class="CmbBox"() -> ("Strings[]"=w252:string[])  [unwired: 2 in, 2 out]
        n122 = Fract/Exp String To Number(string=w242) -> (number=w240:dbl)  [unwired: 3 in, 1 out]
        n123 = Fract/Exp String To Number(string=w243) -> (number=w241:dbl)  [unwired: 3 in, 1 out]
        n124 = local write "generarA2"(TRUE ("generarA_1")) -> ()
        n125 = Index Array(array=w252, index=w246) -> (element=w251:string)
        n126 = Bundle By Name(cluster=w244, "frec"=w241, "amplit"=w240) -> (w239:T1)
        n127 = property on="cb_frec_A_2" class="CmbBox"("Value"=w251) -> ()  [unwired: 2 in, 2 out]
        n128 = Bundle By Name(cluster=T7 {"Estados"=enum."iniciarGEN", "Data"=variant} ("Module Dat Cluster"), "Estados"=Estados."iniciarGEN", "Data"="A2" ("message")) -> (w237:T7)
        n129 = call "Queueu Comms Enqueue.vi"("error in"=w232, "Element"=w237) -> ("error out"=w235:errorcluster)  [unwired: 8 in, 1 out]
      }
      frame "FrecAmp_C2" {
        # "volt"
        # "frec"
        # "cambia el valor del Combo Box"
        # "obtengo \nfrecuencia a generar"
        n130 = Index Array(array=w274, index (dim 0)=1 ("index (page)")) -> (element=w273:string[][])  [unwired: 2 in]
        n131 = Flush Queue(queue=w256, error in (no error)=w258) -> (error out=w257:errorcluster)  [unwired: 2 out]
        n132 = call "FGV_fila.vi"("action"=enum16{"increment", "set_start", "get"}."get") -> ("fila out"=w271:i32)  [unwired: 3 in, 1 out]
        "fila actual C" <- w271
        n133 = Index Array(array=w273, index (row) #1=w271, index (col) #1=0 ("disabled index (col)"), index (row) #2=w271, index (col) #2=1 ("disabled index (col)")) -> (element #1=w268:string, element #2=w267:string)
        "frec_generar_C2" <- w268
        "volt_generar_C2" <- w267
        n134 = property on="cb_frec_C_2" class="CmbBox"() -> ("Strings[]"=w277:string[])  [unwired: 2 in, 2 out]
        n135 = Fract/Exp String To Number(string=w267) -> (number=w265:dbl)  [unwired: 3 in, 1 out]
        n136 = Fract/Exp String To Number(string=w268) -> (number=w266:dbl)  [unwired: 3 in, 1 out]
        n137 = local write "generarC2"(TRUE ("generarA_1")) -> ()
        n138 = Index Array(array=w277, index=w271) -> (element=w276:string)
        n139 = Bundle By Name(cluster=w269, "frec"=w266, "amplit"=w265) -> (w264:T1)
        n140 = property on="cb_frec_C_2" class="CmbBox"("Value"=w276) -> ()  [unwired: 2 in, 2 out]
        n141 = Bundle By Name(cluster=T7 {"Estados"=enum."iniciarGEN", "Data"=variant} ("Module Dat Cluster"), "Estados"=Estados."iniciarGEN", "Data"="C2" ("message")) -> (w262:T7)
        n142 = call "Queueu Comms Enqueue.vi"("error in"=w257, "Element"=w262) -> ("error out"=w260:errorcluster)  [unwired: 8 in, 1 out]
      }
      frame "FrecAmp_Z2" {
        # "volt"
        # "frec"
        # "cambia el valor del Combo Box"
        # "obtengo \nfrecuencia a generar"
        n143 = Index Array(array=w299, index (dim 0)=2 ("index (page)")) -> (element=w298:string[][])  [unwired: 2 in]
        n144 = Flush Queue(queue=w281, error in (no error)=w283) -> (error out=w282:errorcluster)  [unwired: 2 out]
        n145 = call "FGV_fila.vi"("action"=enum16{"increment", "set_start", "get"}."get") -> ("fila out"=w296:i32)  [unwired: 3 in, 1 out]
        "fila actual Z" <- w296
        n146 = Index Array(array=w298, index (row) #1=w296, index (col) #1=0 ("disabled index (col)"), index (row) #2=w296, index (col) #2=1 ("disabled index (col)")) -> (element #1=w293:string, element #2=w292:string)
        "frec_generar_Z2" <- w293
        "volt_generar_Z2" <- w292
        n147 = property on="cb_frec_Z_2" class="CmbBox"() -> ("Strings[]"=w302:string[])  [unwired: 2 in, 2 out]
        n148 = Fract/Exp String To Number(string=w292) -> (number=w290:dbl)  [unwired: 3 in, 1 out]
        n149 = Fract/Exp String To Number(string=w293) -> (number=w291:dbl)  [unwired: 3 in, 1 out]
        n150 = local write "generarZ2"(TRUE ("generarA_1")) -> ()
        n151 = Index Array(array=w302, index=w296) -> (element=w301:string)
        n152 = Bundle By Name(cluster=w294, "frec"=w291, "amplit"=w290) -> (w289:T1)
        n153 = property on="cb_frec_Z_2" class="CmbBox"("Value"=w301) -> ()  [unwired: 2 in, 2 out]
        n154 = Bundle By Name(cluster=T7 {"Estados"=enum."iniciarGEN", "Data"=variant} ("Module Dat Cluster"), "Estados"=Estados."iniciarGEN", "Data"="Z2" ("message")) -> (w287:T7)
        n155 = call "Queueu Comms Enqueue.vi"("error in"=w282, "Element"=w287) -> ("error out"=w285:errorcluster)  [unwired: 8 in, 1 out]
      }
      frame "iniciarGEN" {
        # "Prepara la frec y amplitusd para comenzar\nla generacion de la señal"
        n156 = Variant To Data(error in=w314, type="", Variant=w306) -> (data=w305:string, error out=w308:errorcluster)
        n157 = Unbundle By Name(w312) -> ()  [unwired: 2 out]
        n158 = Bundle By Name(cluster=T7 {"Estados"=enum."monitoreo", "Data"=variant} ("Module Dat Cluster"), "Estados"=Estados."monitoreo", "Data"=w305) -> (w310:T7)
        n159 = call "Queueu Comms Enqueue.vi"("error in"=w308, "Element"=w310) -> ("error out"=w313:errorcluster)  [unwired: 8 in, 1 out]
        "FrecAmpGEN" <- w312
      }
      frame "monitoreo" {
        n160 = Variant To Data(error in=w333, type="", Variant=w324) -> (data=w321:string, error out=w322:errorcluster)
        n161 = Unbundle By Name(w325) -> ("frec"=w327:dbl, "amplit"=w326:dbl)
        n162 = Random Number (0-1)() -> (number: 0 to 1=w332:dbl)
        n163 = Random Number (0-1)() -> (number: 0 to 1=w331:dbl)
        n164 = Add(x=w326, y=w332) -> (x+y=w328:dbl)
        n165 = Add(x=w327, y=w331) -> (x+y=w329:dbl)
        n166 = case shown="\"Z1\"" w321 {
          tunnel: w329 -> [_ w336 w338 w340 w342 w344 w346]
          tunnel: w328 -> [_ w335 w337 w339 w341 w343 w345]
          frame "False", Default {
          }
          frame "A1" {
            "frecMonA_1" <- w336
            "voltMonA_1" <- w335
          }
          frame "A2" {
            "frecMonA_2" <- w338
            "voltMonA_2" <- w337
          }
          frame "C1" {
            "frecMonC_1" <- w340
            "voltMonC_1" <- w339
          }
          frame "C2" {
            "frecMonC_2" <- w342
            "voltMonC_2" <- w341
          }
          frame "Z1" {
            "frecMonZ_1" <- w344
            "voltMonZ_1" <- w343
          }
          frame "Z2" {
            "frecMonZ_2" <- w346
            "voltMonZ_2" <- w345
          }
        }
        n167 = Bundle By Name(cluster=T7 {"Estados"=enum."monitoreo", "Data"=variant} ("Module Dat Cluster"), "Estados"=Estados."monitoreo", "Data"=w321) -> (w320:T7)
        n168 = call "Queueu Comms Enqueue.vi"("error in"=w322, "Element"=w320) -> ("error out"=w317:errorcluster)  [unwired: 8 in, 1 out]
        n169 = Wait (ms)(milliseconds to wait=u32 250) -> ()  [unwired: 1 out]
      }
      frame "detenerGEN" {
        w350 = 0.0 ("frecMonA_1")
        w351 = 0.0 ("frecMonA_1")
        # "comando GPIB para detener la geenracion"
        n170 = Flush Queue(queue=w348, error in (no error)=w353) -> (error out=w349:errorcluster)  [unwired: 2 out]
        n171 = local write "frecMonA_1"(w351) -> ()
        n172 = local write "voltMonA_1"(w351) -> ()
        n173 = local write "voltMonA_2"(w351) -> ()
        n174 = local write "frecMonA_2"(w351) -> ()
        n175 = local write "voltMonC_1"(w351) -> ()
        n176 = local write "frecMonC_1"(w351) -> ()
        n177 = local write "voltMonC_2"(w350) -> ()
        n178 = local write "frecMonC_2"(w350) -> ()
        n179 = local write "voltMonZ_1"(w350) -> ()
        n180 = local write "frecMonZ_1"(w350) -> ()
        n181 = local write "voltMonZ_2"(w350) -> ()
        n182 = local write "frecMonZ_2"(w350) -> ()
      }
      frame "crea_voltajes_prueba_A" {
        w371 = dbl[] [-39.4, -26.2, -16.1, -8.6, -3.2, 0.0, 1.2, 1.0, -1.1, -6.6]  # Ponderaciones_A
        # "Vf1 =(VRef) x 10 ^( Pf1 / 20)\n\nVf1 = Voltaje para frecuencia 1\nVref = Voltaje de referencia según ajuste\nPf1= Ponderación A según Base de datos"
        n183 = property on="cb_frec_A_2" class="CmbBox"() -> ("Value"=→"frec_ref_A":string)  [unwired: 2 in, 2 out]
        n184 = Flush Queue(queue=w357, error in (no error)=w361) -> (error out=w358:errorcluster)  [unwired: 2 out]
        n185 = for {
          tunnel: w371 -> [w380] mode=indexing
          tunnel: [w372] -> w364 mode=indexing
          # "Pfx"
          n186 = local read "Vref_A"() -> (w375:dbl)
          n187 = Divide(x=w380, y=20.0) -> (x/y=w377:dbl)
          n188 = Power Of X(1:10.0 ("x"), 2:w377) -> (0:w376:dbl)
          n189 = Multiply(x=w376, y=w375) -> (x*y=w374:dbl)
          n190 = Number To Fractional String(number=w374, precision (6)=i16 3) -> (F-format string=w372:string)  [unwired: 2 in]
        }
        "Voltajes_Ref_A" <- w364
        n191 = Index Array(array=w367, index (dim 0)=0 ("index (page)")) -> (element=w369:string[][])  [unwired: 2 in]
        n192 = call "escribeEnTabla.vi"("parametros"=w364, "col"=1, "tabla in"=w369) -> ("tabla out"=w365:string[][])  [unwired: 8 in]
        n193 = Replace Array Subset(array=w367, new element=w365, index (dim 0)=0 ("index (page)")) -> (w366:string[][][])  [unwired: 2 in]
        n194 = local write "Tabla_A"(w365) -> ()
        n195 = call "Queueu Comms Enqueue.vi"("error in"=w358, "Element"=T7 {"Estados"=enum."voltajeInicialA2", "Data"=variant} ("Module Dat Cluster")) -> ("error out"=w360:errorcluster)  [unwired: 8 in, 1 out]
      }
      frame "crea_voltajes_prueba_C" {
        w397 = dbl[] [-3.0, -0.8, -0.2, 0.0, 0.0, 0.0, -0.2, -0.8, -3.0, -8.5]  # Ponderaciones_C
        # "Vf1 =(VRef) x 10 ^( Pf1 / 20)\n\nVf1 = Voltaje para frecuencia 1\nVref = Voltaje de referencia según ajuste\nPf1= Ponderación A según Base de datos"
        n196 = property on="cb_frec_C_2" class="CmbBox"() -> ("Value"=→"frec_ref_C":string)  [unwired: 2 in, 2 out]
        n197 = Flush Queue(queue=w384, error in (no error)=w388) -> (error out=w385:errorcluster)  [unwired: 2 out]
        n198 = for {
          tunnel: w397 -> [w406] mode=indexing
          tunnel: [w398] -> w382 mode=indexing
          # "Pfx"
          n199 = local read "Vref_C"() -> (w401:dbl)
          n200 = Divide(x=w406, y=20.0) -> (x/y=w403:dbl)
          n201 = Power Of X(1:10.0 ("x"), 2:w403) -> (0:w402:dbl)
          n202 = Multiply(x=w402, y=w401) -> (x*y=w400:dbl)
          n203 = Number To Fractional String(number=w400, precision (6)=i16 3) -> (F-format string=w398:string)  [unwired: 2 in]
        }
        "Voltajes_Ref_C" <- w382
        n204 = Index Array(array=w393, index (dim 0)=1 ("index (page)")) -> (element=w395:string[][])  [unwired: 2 in]
        n205 = call "escribeEnTabla.vi"("parametros"=w382, "col"=1, "tabla in"=w395) -> ("tabla out"=w391:string[][])  [unwired: 8 in]
        n206 = Replace Array Subset(array=w393, new element=w391, index (dim 0)=1 ("index (page)")) -> (w392:string[][][])  [unwired: 2 in]
        n207 = local write "Tabla_C"(w391) -> ()
        n208 = call "Queueu Comms Enqueue.vi"("error in"=w385, "Element"=T7 {"Estados"=enum."voltajeInicialC2", "Data"=variant} ("Module Dat Cluster")) -> ("error out"=w387:errorcluster)  [unwired: 8 in, 1 out]
      }
      frame "crea_voltajes_prueba_Z" {
        w423 = dbl[] [0.0, 0.0, 0.0, 0.0, 0.0, 0.0, 0.0, 0.0, 0.0, 0.0]  # Ponderaciones_Z
        # "Vf1 =(VRef) x 10 ^( Pf1 / 20)\n\nVf1 = Voltaje para frecuencia 1\nVref = Voltaje de referencia según ajuste\nPf1= Ponderación A según Base de datos"
        n209 = property on="cb_frec_Z_2" class="CmbBox"() -> ("Value"=→"frec_ref_Z_2":string)  [unwired: 2 in, 2 out]
        n210 = Flush Queue(queue=w410, error in (no error)=w414) -> (error out=w411:errorcluster)  [unwired: 2 out]
        n211 = for {
          tunnel: w423 -> [w432] mode=indexing
          tunnel: [w424] -> w407 mode=indexing
          # "Pfx"
          n212 = local read "Vref_Z"() -> (w427:dbl)
          n213 = Divide(x=w432, y=20.0) -> (x/y=w429:dbl)
          n214 = Power Of X(1:10.0 ("x"), 2:w429) -> (0:w428:dbl)
          n215 = Multiply(x=w428, y=w427) -> (x*y=w426:dbl)
          n216 = Number To Fractional String(number=w426, precision (6)=i16 3) -> (F-format string=w424:string)  [unwired: 2 in]
        }
        "Voltajes_Ref_Z" <- w407
        n217 = Index Array(array=w419, index (dim 0)=2 ("index (page)")) -> (element=w421:string[][])  [unwired: 2 in]
        n218 = call "escribeEnTabla.vi"("parametros"=w407, "col"=1, "tabla in"=w421) -> ("tabla out"=w417:string[][])  [unwired: 8 in]
        n219 = Replace Array Subset(array=w419, new element=w417, index (dim 0)=2 ("index (page)")) -> (w418:string[][][])  [unwired: 2 in]
        n220 = local write "Tabla_Z"(w417) -> ()
        n221 = call "Queueu Comms Enqueue.vi"("error in"=w411, "Element"=T7 {"Estados"=enum."voltajeInicialZ2", "Data"=variant} ("Module Dat Cluster")) -> ("error out"=w413:errorcluster)  [unwired: 8 in, 1 out]
      }
      frame "voltajeInicialA2" {
        n222 = local read "Voltajes_Ref_A"() -> (w437:string[])
        n223 = call "FGV_fila.vi"("action"=enum16{"increment", "set_start", "get"}."get") -> ("fila out"=w438:i32)  [unwired: 3 in, 1 out]
        n224 = Index Array(array=w437, index=w438) -> (element=w439:string)
        n225 = Fract/Exp String To Number(string=w439) -> (number=→"voltaje_A":dbl)  [unwired: 3 in, 1 out]
      }
      frame "voltajeInicialC2" {
        n226 = local read "Voltajes_Ref_C"() -> (w447:string[])
        n227 = call "FGV_fila.vi"("action"=enum16{"increment", "set_start", "get"}."get") -> ("fila out"=w448:i32)  [unwired: 3 in, 1 out]
        n228 = Index Array(array=w447, index=w448) -> (element=w449:string)
        n229 = Fract/Exp String To Number(string=w449) -> (number=→"voltaje_C":dbl)  [unwired: 3 in, 1 out]
      }
      frame "voltajeInicialZ2" {
        n230 = local read "Voltajes_Ref_Z"() -> (w457:string[])
        n231 = call "FGV_fila.vi"("error in (no error)"=w452, "action"=enum16{"increment", "set_start", "get"}."get") -> ("error out"=w451:errorcluster, "fila out"=w458:i32)  [unwired: 2 in]
        n232 = Index Array(array=w457, index=w458) -> (element=w459:string)
        n233 = Fract/Exp String To Number(string=w459) -> (number=→"voltaje_Z":dbl)  [unwired: 3 in, 1 out]
      }
      frame "actualizarVrefA" {
        n234 = local read "Voltajes_Ref_A"() -> (w467:string[])
        n235 = call "FGV_fila.vi"("error in (no error)"=w466, "action"=enum16{"increment", "set_start", "get"}."get") -> ("error out"=w465:errorcluster, "fila out"=w464:i32)  [unwired: 2 in]
        n236 = Index Array(array=w467, index=w464) -> (element=w463:string)
        n237 = Fract/Exp String To Number(string=w463, default (0 dbl)=0.0 ("default (0 I32)")) -> (number=w462:dbl)  [unwired: 2 in, 1 out]
        n238 = local write "voltaje_A"(w462) -> ()
      }
      frame "actualizarVrefC" {
        n239 = local read "Voltajes_Ref_C"() -> (w478:string[])
        n240 = call "FGV_fila.vi"("error in (no error)"=w477, "action"=enum16{"increment", "set_start", "get"}."get") -> ("error out"=w476:errorcluster, "fila out"=w475:i32)  [unwired: 2 in]
        n241 = Index Array(array=w478, index=w475) -> (element=w474:string)
        n242 = Fract/Exp String To Number(string=w474, default (0 dbl)=0.0 ("default (0 I32)")) -> (number=w473:dbl)  [unwired: 2 in, 1 out]
        n243 = local write "voltaje_C"(w473) -> ()
      }
      frame "actualizarVrefZ" {
        n244 = local read "Voltajes_Ref_Z"() -> (w489:string[])
        n245 = call "FGV_fila.vi"("error in (no error)"=w488, "action"=enum16{"increment", "set_start", "get"}."get") -> ("error out"=w487:errorcluster, "fila out"=w486:i32)  [unwired: 2 in]
        n246 = Index Array(array=w489, index=w486) -> (element=w485:string)
        n247 = Fract/Exp String To Number(string=w485, default (0 dbl)=0.0 ("default (0 I32)")) -> (number=w484:dbl)  [unwired: 2 in, 1 out]
        n248 = local write "voltaje_Z"(w484) -> ()
      }
      frame "ingresaMedicionesA" {
        n249 = Flush Queue(queue=w494, error in (no error)=w496) -> (error out=w495:errorcluster)  [unwired: 2 out]
        n250 = Index Array(array=w513, index (dim 0)=0 ("index (page)")) -> (element=w500:string[][])  [unwired: 2 in]
        n251 = Variant To Data(error in=w495, type=string[][] [] ("NewVal"), Variant=w515) -> (data=w502:string[][], error out=w504:errorcluster)
        n252 = control-ref of="Tabla_A"() -> (w499:refnum<vi>)
        n253 = call "ingresaMediciones.vi"("New Value"=w502, "Tbl Refnum"=w499, "error in (no error)"=w504, "mediciones in"=w501, "Tabla in"=w500) -> ("error out"=w503:errorcluster, "mediciones out"=w497:T9, "Tabla out"=w498:string[][])  [unwired: 3 in, 1 out]
        n254 = Replace Array Subset(array=w513, new element=w498, index (dim 0)=0 ("index (page)")) -> (w512:string[][][])  [unwired: 2 in]
        n255 = Bundle By Name(cluster=T7 {"Estados"=enum."ingresaMedicionesA", "Data"=variant} ("Element"), "Estados"=Estados."cumplimiento", "Data"="A") -> (w507:T7)
        n256 = call "Queueu Comms Enqueue.vi"("error in"=w503, "Element"=w507) -> ("error out"=w510:errorcluster)  [unwired: 8 in, 1 out]
      }
      frame "ingresaMedicionesC" {
        n257 = Flush Queue(queue=w517, error in (no error)=w519) -> (error out=w518:errorcluster)  [unwired: 2 out]
        n258 = Index Array(array=w536, index (dim 0)=1 ("index (page)")) -> (element=w523:string[][])  [unwired: 2 in]
        n259 = Variant To Data(error in=w518, type=string[][] [] ("NewVal"), Variant=w538) -> (data=w525:string[][], error out=w527:errorcluster)
        n260 = control-ref of="Tabla_C"() -> (w522:refnum<vi>)
        n261 = call "ingresaMediciones.vi"("New Value"=w525, "Tbl Refnum"=w522, "error in (no error)"=w527, "mediciones in"=w524, "Tabla in"=w523) -> ("error out"=w526:errorcluster, "mediciones out"=w520:T9, "Tabla out"=w521:string[][])  [unwired: 3 in, 1 out]
        n262 = Replace Array Subset(array=w536, new element=w521, index (dim 0)=1 ("index (page)")) -> (w535:string[][][])  [unwired: 2 in]
        n263 = Bundle By Name(cluster=T7 {"Estados"=enum."ingresaMedicionesA", "Data"=variant} ("Element"), "Estados"=Estados."cumplimiento", "Data"="C") -> (w530:T7)
        n264 = call "Queueu Comms Enqueue.vi"("error in"=w526, "Element"=w530) -> ("error out"=w533:errorcluster)  [unwired: 8 in, 1 out]
      }
      frame "ingresaMedicionesZ" {
        n265 = Flush Queue(queue=w540, error in (no error)=w542) -> (error out=w541:errorcluster)  [unwired: 2 out]
        n266 = Index Array(array=w559, index (dim 0)=2 ("index (page)")) -> (element=w546:string[][])  [unwired: 2 in]
        n267 = Variant To Data(error in=w541, type=string[][] [] ("NewVal"), Variant=w561) -> (data=w548:string[][], error out=w550:errorcluster)
        n268 = control-ref of="Tabla_Z"() -> (w545:refnum<vi>)
        n269 = call "ingresaMediciones.vi"("New Value"=w548, "Tbl Refnum"=w545, "error in (no error)"=w550, "mediciones in"=w547, "Tabla in"=w546) -> ("error out"=w549:errorcluster, "mediciones out"=w543:T9, "Tabla out"=w544:string[][])  [unwired: 3 in, 1 out]
        n270 = Replace Array Subset(array=w559, new element=w544, index (dim 0)=2 ("index (page)")) -> (w558:string[][][])  [unwired: 2 in]
        n271 = Bundle By Name(cluster=T7 {"Estados"=enum."ingresaMedicionesA", "Data"=variant} ("Element"), "Estados"=Estados."cumplimiento", "Data"="Z") -> (w553:T7)
        n272 = call "Queueu Comms Enqueue.vi"("error in"=w549, "Element"=w553) -> ("error out"=w556:errorcluster)  [unwired: 8 in, 1 out]
      }
      frame "cumplimiento" {
        n273 = Variant To Data(error in=w579, type="", Variant=w578) -> (data=w566:string, error out=w577:errorcluster)
        n274 = case shown="\"Z\"" w566 {
          tunnel: [0 ("index (page)") 1 ("index (page)") 2 ("index (page)")] -> w564
          frame "A", Default {
          }
          frame "C" {
          }
          frame "Z" {
          }
        }
        n275 = Index Array(array=w576, index (dim 0)=w564) -> (element=w575:string[][])  [unwired: 2 in]
        n276 = call "cumplimiento.vi"("error in (no error)"=w577, "mediciones in"=w574, "Tabla in"=w575) -> ("error out"=w567:errorcluster, "mediciones out"=w573:T9, "Tabla out"=w565:string[][])  [unwired: 5 in, 1 out]
        n277 = Replace Array Subset(array=w576, new element=w565, index (dim 0)=w564) -> (w572:string[][][])  [unwired: 2 in]
        n278 = case shown="2" w564 {
          tunnel: w565 -> [w583 w585 _ w588]
          tunnel: ["C2" "Z2" "" "A2"] -> w563
          frame 1 {
            n279 = local write "Tabla_C"(w583) -> ()
          }
          frame 2 {
            n280 = local write "Tabla_Z"(w585) -> ()
          }
          frame Default {
          }
          frame 0 {
            n281 = local write "Tabla_A"(w588) -> ()
          }
        }
        n282 = Bundle By Name(cluster=T7 {"Estados"=enum."ingresaMedicionesA", "Data"=variant} ("Element"), "Estados"=Estados."listo_evaluar", "Data"=w563) -> (w571:T7)
        n283 = call "Queueu Comms Enqueue.vi"("error in"=w567, "Element"=w571) -> ("error out"=w568:errorcluster)  [unwired: 8 in, 1 out]
      }
      frame "listo_evaluar" {
        # "si son todos\ndistntos a cero\nentonces todos se\nhan evaluado"
        n284 = Variant To Data(error in=w600, type="" ("y"), Variant=w594) -> (data=w592:string, error out=w595:errorcluster)
        n285 = case shown="\"C2\"" w592 {
          tunnel: w597 -> [w612 w630 w648]
          tunnel: [w610 w628 w646] -> w596
          tunnel: w595 -> [w603 w621 w639]
          frame "A2", Default {
            n286 = Index Array(array=w612, index (dim 0)=0 ("index (page)")) -> (element=w611:string[][])  [unwired: 2 in]
            n287 = Index Array(array=w611, index (col)=8 ("disabled index (col)")) -> (element=w614:string[])  [unwired: 1 in]
            n288 = for {
              tunnel: [w618] -> w613 mode=indexing
              tunnel: w614 -> [w616] mode=indexing
              n289 = Not Equal?(x=w616, y="") -> (x != y?=w618:bool)
            }
            n290 = And Array Elements(Boolean array=w613) -> (logical AND=w609:bool)
            n291 = Select(t=Estados."evaluar" ("Estados"), s=w609, f=Estados."monitoreo" ("Estados")) -> (s? t:f=w605:T8)
            n292 = Bundle By Name(cluster=T7 {"Estados"=enum."salir", "Data"=variant} ("Element"), "Estados"=w605, "Data"="A2" ("y")) -> (w604:T7)
            n293 = call "Queueu Comms Enqueue.vi"("error in"=w603, "Element"=w604) -> ("error out"=w610:errorcluster)  [unwired: 8 in, 1 out]
          }
          frame "C2" {
            n294 = Index Array(array=w630, index (dim 0)=1 ("index (page)")) -> (element=w629:string[][])  [unwired: 2 in]
            n295 = Index Array(array=w629, index (col)=8 ("disabled index (col)")) -> (element=w632:string[])  [unwired: 1 in]
            n296 = for {
              tunnel: [w636] -> w631 mode=indexing
              tunnel: w632 -> [w634] mode=indexing
              n297 = Not Equal?(x=w634, y="") -> (x != y?=w636:bool)
            }
            n298 = And Array Elements(Boolean array=w631) -> (logical AND=w627:bool)
            n299 = Select(t=Estados."evaluar" ("Estados"), s=w627, f=Estados."monitoreo" ("Estados")) -> (s? t:f=w623:T8)
            n300 = Bundle By Name(cluster=T7 {"Estados"=enum."salir", "Data"=variant} ("Element"), "Estados"=w623, "Data"="C2" ("y")) -> (w622:T7)
            n301 = call "Queueu Comms Enqueue.vi"("error in"=w621, "Element"=w622) -> ("error out"=w628:errorcluster)  [unwired: 8 in, 1 out]
          }
          frame "Z2" {
            n302 = Index Array(array=w648, index (dim 0)=2 ("index (page)")) -> (element=w647:string[][])  [unwired: 2 in]
            n303 = Index Array(array=w647, index (col)=8 ("disabled index (col)")) -> (element=w650:string[])  [unwired: 1 in]
            n304 = for {
              tunnel: [w654] -> w649 mode=indexing
              tunnel: w650 -> [w652] mode=indexing
              n305 = Not Equal?(x=w652, y="") -> (x != y?=w654:bool)
            }
            n306 = And Array Elements(Boolean array=w649) -> (logical AND=w645:bool)
            n307 = Select(t=Estados."evaluar" ("Estados"), s=w645, f=Estados."monitoreo" ("Estados")) -> (s? t:f=w641:T8)
            n308 = Bundle By Name(cluster=T7 {"Estados"=enum."salir", "Data"=variant} ("Element"), "Estados"=w641, "Data"="Z2" ("y")) -> (w640:T7)
            n309 = call "Queueu Comms Enqueue.vi"("error in"=w639, "Element"=w640) -> ("error out"=w646:errorcluster)  [unwired: 8 in, 1 out]
          }
        }
      }
      frame "evaluar" {
        n310 = Variant To Data(error in=w664, type="" ("y"), Variant=w656) -> (data=w655:string, error out=w658:errorcluster)
        n311 = case shown="\"Z2\"" w655 {
          tunnel: w661 -> [_ w667 w677 w687]
          frame "False", Default {
          }
          frame "A2" {
            # "si todos cumpln\nentonces el ensayo\ncumple"
            n312 = Index Array(array=w667, index (dim 0)=0 ("index (page)")) -> (element=w666:string[][])  [unwired: 2 in]
            n313 = Index Array(array=w666, index (col)=8 ("disabled index (col)")) -> (element=w669:string[])  [unwired: 1 in]
            n314 = for {
              tunnel: [w674] -> w670 mode=indexing
              tunnel: w669 -> [w672] mode=indexing
              n315 = Equal?(x=w672, y="Cumple") -> (x = y?=w674:bool)
            }
            n316 = And Array Elements(Boolean array=w670) -> (logical AND=→"cumple_no_cumple_A":bool)
          }
          frame "C2" {
            # "si todos cumpln\nentonces el ensayo\ncumple"
            n317 = Index Array(array=w677, index (dim 0)=1 ("index (page)")) -> (element=w676:string[][])  [unwired: 2 in]
            n318 = Index Array(array=w676, index (col)=8 ("disabled index (col)")) -> (element=w679:string[])  [unwired: 1 in]
            n319 = for {
              tunnel: [w684] -> w680 mode=indexing
              tunnel: w679 -> [w682] mode=indexing
              n320 = Equal?(x=w682, y="Cumple") -> (x = y?=w684:bool)
            }
            n321 = And Array Elements(Boolean array=w680) -> (logical AND=→"cumple_no_cumple_C":bool)
          }
          frame "Z2" {
            # "si todos cumpln\nentonces el ensayo\ncumple"
            n322 = Index Array(array=w687, index (dim 0)=2 ("index (page)")) -> (element=w686:string[][])  [unwired: 2 in]
            n323 = Index Array(array=w686, index (col)=8 ("disabled index (col)")) -> (element=w689:string[])  [unwired: 1 in]
            n324 = for {
              tunnel: [w694] -> w690 mode=indexing
              tunnel: w689 -> [w692] mode=indexing
              n325 = Equal?(x=w692, y="Cumple") -> (x = y?=w694:bool)
            }
            n326 = And Array Elements(Boolean array=w690) -> (logical AND=→"cumple_no_cumple_Z":bool)
          }
        }
        n327 = call "Queueu Comms Enqueue.vi"("error in"=w658, "Element"=T7 {"Estados"=enum."final", "Data"=variant}) -> ("error out"=w660:errorcluster)  [unwired: 8 in, 1 out]
      }
      frame "final" {
        n328 = local read "cumple_no_cumple_A"() -> (w699:bool)
        "cumple_A" <- w699
        n329 = Not(x=w699) -> (.not. x?=→"no_cumple_A":bool)
        n330 = local read "cumple_no_cumple_Z"() -> (w696:bool)
        "cumple_Z" <- w696
        n331 = local read "cumple_no_cumple_C"() -> (w698:bool)
        "cumple_C" <- w698
        n332 = Not(x=w696) -> (.not. x?=→"no_cumple_Z":bool)
        n333 = Not(x=w698) -> (.not. x?=→"no_cumple_C":bool)
      }
      frame "guardaMedicionesA" {
        # "error"
        # "10"
        # "n° filas"
        n334 = Index Array(array=w730, index (dim 0)=0 ("index (page)")) -> (element=w716:string[][])  [unwired: 2 in]
        n335 = local write "generarA2"(FALSE ("generar_A_2")) -> ()
        n336 = call "FGV_fila.vi"("action"=enum16{"increment", "set_start", "get"}."get") -> ("fila out"=w726:i32)  [unwired: 3 in, 1 out]
        n337 = Unbundle By Name(w709) -> ("Medido"=w725:dbl, "Ref"=w724:dbl)
        n338 = property on="cb_frec_A_2" class="CmbBox"() -> ("Strings[]"=w733:string[])  [unwired: 2 in, 2 out]
        n339 = call "FGV_fila.vi"("action"=enum16{"increment", "set_start", "get"}."increment") -> ("fila out"=w715:i32)  [unwired: 3 in, 1 out]
        n340 = Subtract(x=w725, y=w724) -> (x-y=w708:dbl)
        n341 = Equal?(x=w725, y=0.0) -> (x = y?=w722:bool)
        n342 = case shown="True" w722 {
          frame False {
          }
          frame True {
            n343 = One Button Dialog(message="Ingrese valor medido") -> ()  [unwired: 1 in, 1 out]
          }
        }
        n344 = Index Array(array=w716, index (row)=w715, index (col)=1 ("disabled index (col)")) -> (element=w714:string)
        n345 = Index Array(array=w733, index=w715) -> (element=w734:string)
        n346 = Fract/Exp String To Number(string=w714) -> (number=w735:dbl)  [unwired: 3 in, 1 out]
        n347 = call "escribeEnTablaUnValor.vi"("element"=w708, "fila"=w726, "col"=4, "tabla in"=w716) -> ("tabla out"=w719:string[][])  [unwired: 7 in]
        n348 = property on="cb_frec_A_2" class="CmbBox"("Value"=w734) -> ()  [unwired: 2 in, 2 out]
        n349 = local write "voltaje_A"(w735) -> ()
        n350 = Matrix Size(0:w719) -> (1:w718:i32)  [unwired: 1 out]
        n351 = Bundle By Name(cluster=w709, "Medido"=0.0) -> (w707:T4)
        n352 = Decrement(x=w718) -> (x-1=w717:i32)
        n353 = Replace Array Subset(array=w730, new element=w719, index (dim 0)=0 ("index (page)")) -> (w729:string[][][])  [unwired: 2 in]
        n354 = Less?(x=w717, y=w715) -> (x < y?=w710:bool)
        n355 = case shown="True" w710 {
          tunnel: w712 -> [w738 w741]
          tunnel: [w737 w740] -> w711
          frame False {
            n356 = call "Queueu Comms Enqueue.vi"("error in"=w738, "Element"=T7 {"Estados"=enum."detenerGEN", "Data"=variant}) -> ("error out"=w737:errorcluster)  [unwired: 8 in, 1 out]
          }
          frame True {
            n357 = call "Queueu Comms Enqueue.vi"("error in"=w741, "Element"=T7 {"Estados"=enum."ultimaFrec", "Data"=variant}) -> ("error out"=w740:errorcluster)  [unwired: 8 in, 1 out]
          }
        }
      }
      frame "guardaMedicionesC" {
        # "error"
        # "10"
        # "n° filas"
        n358 = Index Array(array=w768, index (dim 0)=1 ("index (page)")) -> (element=w754:string[][])  [unwired: 2 in]
        n359 = local write "generarC2"(FALSE ("generar_A_2")) -> ()
        n360 = call "FGV_fila.vi"("action"=enum16{"increment", "set_start", "get"}."get") -> ("fila out"=w764:i32)  [unwired: 3 in, 1 out]
        n361 = Unbundle By Name(w747) -> ("Medido"=w763:dbl, "Ref"=w762:dbl)
        n362 = property on="cb_frec_C_2" class="CmbBox"() -> ("Strings[]"=w771:string[])  [unwired: 2 in, 2 out]
        n363 = call "FGV_fila.vi"("action"=enum16{"increment", "set_start", "get"}."increment") -> ("fila out"=w753:i32)  [unwired: 3 in, 1 out]
        n364 = Subtract(x=w763, y=w762) -> (x-y=w746:dbl)
        n365 = Equal?(x=w763, y=0.0) -> (x = y?=w760:bool)
        n366 = case shown="True" w760 {
          frame False {
          }
          frame True {
            n367 = One Button Dialog(message="Ingrese valor medido") -> ()  [unwired: 1 in, 1 out]
          }
        }
        n368 = Index Array(array=w754, index (row)=w753, index (col)=1 ("disabled index (col)")) -> (element=w752:string)
        n369 = Index Array(array=w771, index=w753) -> (element=w772:string)
        n370 = Fract/Exp String To Number(string=w752) -> (number=w773:dbl)  [unwired: 3 in, 1 out]
        n371 = call "escribeEnTablaUnValor.vi"("element"=w746, "fila"=w764, "col"=4, "tabla in"=w754) -> ("tabla out"=w757:string[][])  [unwired: 7 in]
        n372 = property on="cb_frec_C_2" class="CmbBox"("Value"=w772) -> ()  [unwired: 2 in, 2 out]
        n373 = local write "voltaje_C"(w773) -> ()
        n374 = Matrix Size(0:w757) -> (1:w756:i32)  [unwired: 1 out]
        n375 = Bundle By Name(cluster=w747, "Medido"=0.0) -> (w745:T4)
        n376 = Decrement(x=w756) -> (x-1=w755:i32)
        n377 = Replace Array Subset(array=w768, new element=w757, index (dim 0)=1 ("index (page)")) -> (w767:string[][][])  [unwired: 2 in]
        n378 = Less?(x=w755, y=w753) -> (x < y?=w748:bool)
        n379 = case shown="True" w748 {
          tunnel: w750 -> [w776 w779]
          tunnel: [w775 w778] -> w749
          frame False {
            n380 = call "Queueu Comms Enqueue.vi"("error in"=w776, "Element"=T7 {"Estados"=enum."detenerGEN", "Data"=variant}) -> ("error out"=w775:errorcluster)  [unwired: 8 in, 1 out]
          }
          frame True {
            n381 = call "Queueu Comms Enqueue.vi"("error in"=w779, "Element"=T7 {"Estados"=enum."ultimaFrec", "Data"=variant}) -> ("error out"=w778:errorcluster)  [unwired: 8 in, 1 out]
          }
        }
      }
      frame "guardaMedicionesZ" {
        # "error"
        # "10"
        # "n° filas"
        n382 = Index Array(array=w806, index (dim 0)=2 ("index (page)")) -> (element=w792:string[][])  [unwired: 2 in]
        n383 = local write "generarZ2"(FALSE ("generar_A_2")) -> ()
        n384 = call "FGV_fila.vi"("action"=enum16{"increment", "set_start", "get"}."get") -> ("fila out"=w802:i32)  [unwired: 3 in, 1 out]
        n385 = Unbundle By Name(w785) -> ("Medido"=w801:dbl, "Ref"=w800:dbl)
        n386 = property on="cb_frec_Z_2" class="CmbBox"() -> ("Strings[]"=w809:string[])  [unwired: 2 in, 2 out]
        n387 = call "FGV_fila.vi"("action"=enum16{"increment", "set_start", "get"}."increment") -> ("fila out"=w791:i32)  [unwired: 3 in, 1 out]
        n388 = Subtract(x=w801, y=w800) -> (x-y=w784:dbl)
        n389 = Equal?(x=w801, y=0.0) -> (x = y?=w798:bool)
        n390 = case shown="True" w798 {
          frame False {
          }
          frame True {
            n391 = One Button Dialog(message="Ingrese valor medido") -> ()  [unwired: 1 in, 1 out]
          }
        }
        n392 = Index Array(array=w792, index (row)=w791, index (col)=1 ("disabled index (col)")) -> (element=w790:string)
        n393 = Index Array(array=w809, index=w791) -> (element=w810:string)
        n394 = Fract/Exp String To Number(string=w790) -> (number=w811:dbl)  [unwired: 3 in, 1 out]
        n395 = call "escribeEnTablaUnValor.vi"("element"=w784, "fila"=w802, "col"=4, "tabla in"=w792) -> ("tabla out"=w795:string[][])  [unwired: 7 in]
        n396 = property on="cb_frec_Z_2" class="CmbBox"("Value"=w810) -> ()  [unwired: 2 in, 2 out]
        n397 = local write "voltaje_Z"(w811) -> ()
        n398 = Matrix Size(0:w795) -> (1:w794:i32)  [unwired: 1 out]
        n399 = Bundle By Name(cluster=w785, "Medido"=0.0) -> (w783:T4)
        n400 = Decrement(x=w794) -> (x-1=w793:i32)
        n401 = Replace Array Subset(array=w806, new element=w795, index (dim 0)=2 ("index (page)")) -> (w805:string[][][])  [unwired: 2 in]
        n402 = Less?(x=w793, y=w791) -> (x < y?=w786:bool)
        n403 = case shown="True" w786 {
          tunnel: w788 -> [w814 w817]
          tunnel: [w813 w816] -> w787
          frame False {
            n404 = call "Queueu Comms Enqueue.vi"("error in"=w814, "Element"=T7 {"Estados"=enum."detenerGEN", "Data"=variant}) -> ("error out"=w813:errorcluster)  [unwired: 8 in, 1 out]
          }
          frame True {
            n405 = call "Queueu Comms Enqueue.vi"("error in"=w817, "Element"=T7 {"Estados"=enum."ultimaFrec", "Data"=variant}) -> ("error out"=w816:errorcluster)  [unwired: 8 in, 1 out]
          }
        }
      }
      frame "ultimaFrec" {
        n406 = call "FGV_fila.vi"("error in (no error)"=w820, "fila_inicial"=0, "action"=enum16{"increment", "set_start", "get"}."set_start") -> ("error out"=w819:errorcluster)  [unwired: 1 in, 1 out]
        n407 = call "Queueu Comms Enqueue.vi"("error in"=w819, "Element"=T7 {"Estados"=enum."detenerGEN", "Data"=variant} ("Module Dat Cluster")) -> ("error out"=w824:errorcluster)  [unwired: 8 in, 1 out]
        n408 = One Button Dialog(message="Ultima frecuencia") -> ()  [unwired: 1 in, 1 out]
      }
      frame "salir" {
      }
      frame Default {
        n409 = One Button Dialog(message="mensaje equivocado") -> ()  [unwired: 1 in, 1 out]
      }
    }
    n410 = Unbundle By Name(w43) -> ("status"=w42:bool)
    n411 = Or(x=w42, y=w41) -> (x .or. y?=w40:bool)
  }
  n412 = while {
    tunnel: w21 -> [w839]
    tunnel: [w840] -> w20
    stop <- w841 stop-if-true
    n413 = event shown="[6] \"generarA2\": Value Change" {
      selector: _ -> [_ _ _ _ _ _ _ _ _ _ _ _ _ _ _ _ _ _ _ _ _ _ _ _ _ _ _ _]
      dyn-events: _ -> [_ _ _ _ _ _ _ _ _ _ _ _ _ _ _ _ _ _ _ _ _ _ _ _ _ _ _ _]
      timeout: _ -> [_ _ _ _ _ _ _ _ _ _ _ _ _ _ _ _ _ _ _ _ _ _ _ _ _ _ _ _]
      tunnel: [_ _ _ _ _ _ _ _ _ _ _ _ _ _ _ _ _ _ _ _ _ TRUE _ _ _ _ _ _] -> w841
      tunnel: [w842 w845 w848 w860 w873 w886 w891 w902 w913 w924 w927 w930 w935 w939 w943 w944 w950 w954 w961 w968 w975 w980 w991 w997 w1003 w1011 w1021 w1031] -> w840
      tunnel: w839 -> [w843 w846 w849 w852 w865 w878 w895 w906 w917 w923 w926 w929 w934 w938 w942 w945 w949 w957 w964 w971 w977 w979 w992 w998 w1004 w1006 w1017 w1027]
      event "go_A": Value Change {
        # "solo cambia el TAB"
        n414 = event-data() -> ()  [unwired: 1 in, 1 out]
        n415 = property on="Tab" class="TabCtl (strict)"(error in=w843, "Value"=T2."Page 2" ("Tab_Prueba04")) -> (error out=w842:errorcluster)  [unwired: 1 in, 1 out]
      }
      event "go_C": Value Change {
        # "solo cambia el TAB"
        n416 = event-data() -> ()  [unwired: 1 in, 1 out]
        n417 = property on="Tab" class="TabCtl (strict)"(error in=w846, "Value"=T2."Page 4" ("Tab_Prueba04")) -> (error out=w845:errorcluster)  [unwired: 1 in, 1 out]
      }
      event "go_Z": Value Change {
        n418 = event-data() -> ()  [unwired: 1 in, 1 out]
        n419 = property on="Tab" class="TabCtl (strict)"(error in=w849, "Value"=T2."Page 6" ("Tab_Prueba04")) -> (error out=w848:errorcluster)  [unwired: 1 in, 1 out]
      }
      event "generarA1": Value Change {
        n420 = event-data() -> ("NewVal"=w863:bool)  [unwired: 1 in]
        n421 = Equal?(x=w863, y=TRUE) -> (x = y?=w861:bool)
        n422 = property on="VoltAjuste_A" class="Slide (strict)"(error in=w852, "DisabledEnum"=T6."Enabled" ("Disabled")) -> (error out=w851:errorcluster)  [unwired: 1 in, 1 out]
        n423 = Select(t=Estados."FrecAmp_A1" ("Estados"), s=w861, f=Estados."detenerGEN" ("Estados")) -> (s? t:f=w855:T8)
        n424 = Bundle By Name(cluster=T7 {"Estados"=enum."iniciarGEN", "Data"=variant} ("Module Dat Cluster"), "Estados"=w855, "Data"="A1" ("message")) -> (w858:T7)
        n425 = call "Queueu Comms Enqueue.vi"("error in"=w851, "Element"=w858) -> ("error out"=w860:errorcluster)  [unwired: 8 in, 1 out]
      }
      event "generarC1": Value Change {
        n426 = event-data() -> ("NewVal"=w876:bool)  [unwired: 1 in]
        n427 = Equal?(x=w876, y=TRUE) -> (x = y?=w874:bool)
        n428 = property on="VoltAjuste_C" class="Slide (strict)"(error in=w865, "DisabledEnum"=T6."Enabled" ("Disabled")) -> (error out=w864:errorcluster)  [unwired: 1 in, 1 out]
        n429 = Select(t=Estados."FrecAmp_C1" ("Estados"), s=w874, f=Estados."detenerGEN" ("Estados")) -> (s? t:f=w868:T8)
        n430 = Bundle By Name(cluster=T7 {"Estados"=enum."iniciarGEN", "Data"=variant} ("Module Dat Cluster"), "Estados"=w868, "Data"="C1" ("message")) -> (w871:T7)
        n431 = call "Queueu Comms Enqueue.vi"("error in"=w864, "Element"=w871) -> ("error out"=w873:errorcluster)  [unwired: 8 in, 1 out]
      }
      event "generarZ1": Value Change {
        n432 = event-data() -> ("NewVal"=w889:bool)  [unwired: 1 in]
        n433 = Equal?(x=w889, y=TRUE) -> (x = y?=w887:bool)
        n434 = property on="VoltAjuste_Z" class="Slide (strict)"(error in=w878, "DisabledEnum"=T6."Enabled" ("Disabled")) -> (error out=w877:errorcluster)  [unwired: 1 in, 1 out]
        n435 = Select(t=Estados."FrecAmp_Z1" ("Estados"), s=w887, f=Estados."detenerGEN" ("Estados")) -> (s? t:f=w881:T8)
        n436 = Bundle By Name(cluster=T7 {"Estados"=enum."iniciarGEN", "Data"=variant} ("Module Dat Cluster"), "Estados"=w881, "Data"="Z1" ("message")) -> (w884:T7)
        n437 = call "Queueu Comms Enqueue.vi"("error in"=w877, "Element"=w884) -> ("error out"=w886:errorcluster)  [unwired: 8 in, 1 out]
      }
      event "generarA2": Value Change {
        n438 = event-data() -> ("NewVal"=w900:bool)  [unwired: 1 in]
        n439 = Equal?(x=w900, y=TRUE) -> (x = y?=w890:bool)
        n440 = Select(t=Estados."FrecAmp_A2" ("Estados"), s=w890, f=Estados."guardaMedicionesA" ("Estados")) -> (s? t:f=w898:T8)
        n441 = Bundle By Name(cluster=T7 {"Estados"=enum."iniciarGEN", "Data"=variant} ("Module Dat Cluster"), "Estados"=w898, "Data"="A2" ("message")) -> (w893:T7)
        n442 = call "Queueu Comms Enqueue.vi"("error in"=w895, "Element"=w893) -> ("error out"=w891:errorcluster)  [unwired: 8 in, 1 out]
      }
      event "generarC2": Value Change {
        n443 = event-data() -> ("NewVal"=w911:bool)  [unwired: 1 in]
        n444 = Equal?(x=w911, y=TRUE) -> (x = y?=w901:bool)
        n445 = Select(t=Estados."FrecAmp_C2" ("Estados"), s=w901, f=Estados."guardaMedicionesC" ("Estados")) -> (s? t:f=w909:T8)
        n446 = Bundle By Name(cluster=T7 {"Estados"=enum."iniciarGEN", "Data"=variant} ("Module Dat Cluster"), "Estados"=w909, "Data"="C2" ("message")) -> (w904:T7)
        n447 = call "Queueu Comms Enqueue.vi"("error in"=w906, "Element"=w904) -> ("error out"=w902:errorcluster)  [unwired: 8 in, 1 out]
      }
      event "generarZ2": Value Change {
        n448 = event-data() -> ("NewVal"=w922:bool)  [unwired: 1 in]
        n449 = Equal?(x=w922, y=TRUE) -> (x = y?=w912:bool)
        n450 = Select(t=Estados."FrecAmp_Z2" ("Estados"), s=w912, f=Estados."guardaMedicionesZ" ("Estados")) -> (s? t:f=w920:T8)
        n451 = Bundle By Name(cluster=T7 {"Estados"=enum."iniciarGEN", "Data"=variant} ("Module Dat Cluster"), "Estados"=w920, "Data"="Z2" ("message")) -> (w915:T7)
        n452 = call "Queueu Comms Enqueue.vi"("error in"=w917, "Element"=w915) -> ("error out"=w913:errorcluster)  [unwired: 8 in, 1 out]
      }
      event "guardar_Vref_A": Value Change {
        n453 = event-data() -> ()  [unwired: 1 in, 1 out]
        n454 = call "Queueu Comms Enqueue.vi"("error in"=w923, "Element"=T7 {"Estados"=enum."guardarVrefA", "Data"=variant} ("Module Dat Cluster")) -> ("error out"=w924:errorcluster)  [unwired: 8 in, 1 out]
      }
      event "guardar_Vref_C": Value Change {
        n455 = event-data() -> ()  [unwired: 1 in, 1 out]
        n456 = call "Queueu Comms Enqueue.vi"("error in"=w926, "Element"=T7 {"Estados"=enum."guardarVrefC", "Data"=variant} ("Module Dat Cluster")) -> ("error out"=w927:errorcluster)  [unwired: 8 in, 1 out]
      }
      event "guardar_Vref_Z": Value Change {
        n457 = event-data() -> ()  [unwired: 1 in, 1 out]
        n458 = call "Queueu Comms Enqueue.vi"("error in"=w929, "Element"=T7 {"Estados"=enum."guardarVrefZ", "Data"=variant} ("Module Dat Cluster")) -> ("error out"=w930:errorcluster)  [unwired: 8 in, 1 out]
      }
      event Value Change {
        n459 = event-data() -> ()  [unwired: 1 in, 1 out]
        n460 = call "Queueu Comms Enqueue.vi"("error in"=w934, "Element"=T7 {"Estados"=enum."FrecAmp_A1", "Data"=variant}) -> ("error out"=w935:errorcluster)  [unwired: 8 in, 1 out]
        "IndicadorAjuste_A" <- "VoltAjuste_A"
      }
      event Value Change {
        n461 = event-data() -> ()  [unwired: 1 in, 1 out]
        n462 = call "Queueu Comms Enqueue.vi"("error in"=w938, "Element"=T7 {"Estados"=enum."FrecAmp_C1", "Data"=variant}) -> ("error out"=w939:errorcluster)  [unwired: 8 in, 1 out]
        "IndicadorAjuste_C" <- "VoltAjuste_C"
      }
      event Value Change {
        n463 = event-data() -> ()  [unwired: 1 in, 1 out]
        n464 = call "Queueu Comms Enqueue.vi"("error in"=w942, "Element"=T7 {"Estados"=enum."FrecAmp_Z1", "Data"=variant}) -> ("error out"=w943:errorcluster)  [unwired: 8 in, 1 out]
        "IndicadorAjuste_Z" <- "VoltAjuste_Z"
      }
      event "ir a resultados_A": Value Change {
        # "solo cambia el TAB"
        n465 = event-data() -> ()  [unwired: 1 in, 1 out]
        n466 = property on="Tab" class="TabCtl (strict)"("Value"=T2."Page 3" ("Tab_Prueba04")) -> ()  [unwired: 2 in, 2 out]
        n467 = call "Queueu Comms Enqueue.vi"("error in"=w945, "Element"=T7 {"Estados"=enum."crea_voltajes_prueba_A", "Data"=variant} ("Module Dat Cluster")) -> ("error out"=w944:errorcluster)  [unwired: 8 in, 1 out]
      }
      event "ir a resultados_C": Value Change {
        n468 = event-data() -> ()  [unwired: 1 in, 1 out]
        n469 = property on="Tab" class="TabCtl (strict)"(error in=w949, "Value"=T2."Page 5" ("Tab_Prueba04")) -> (error out=w948:errorcluster)  [unwired: 1 in, 1 out]
        n470 = call "Queueu Comms Enqueue.vi"("error in"=w948, "Element"=T7 {"Estados"=enum."crea_voltajes_prueba_C", "Data"=variant} ("Module Dat Cluster")) -> ("error out"=w950:errorcluster)  [unwired: 8 in, 1 out]
      }
      event "ir a inicio desde A": Value Change {
        w958 = TRUE ("ponderacion_A")
        n471 = event-data() -> ()  [unwired: 1 in, 1 out]
        n472 = property on="Tab" class="TabCtl (strict)"(error in=w957, "Value"=T2."Page 1" ("Tab_Prueba04")) -> (error out=w956:errorcluster)  [unwired: 1 in, 1 out]
        n473 = property on="estado_ensayo_A" class="Str"(error in=w956, "Visible"=w958) -> (error out=w955:errorcluster)  [unwired: 1 in, 1 out]
        n474 = call "Queueu Comms Enqueue.vi"("error in"=w955, "Element"=T7 {"Estados"=enum."inicio", "Data"=variant}) -> ("error out"=w954:errorcluster)  [unwired: 8 in, 1 out]
        "ponderacion_A" <- w958
      }
      event "ir a inicio desde C": Value Change {
        w965 = TRUE ("ponderacion_A")
        n475 = event-data() -> ()  [unwired: 1 in, 1 out]
        n476 = property on="Tab" class="TabCtl (strict)"(error in=w964, "Value"=T2."Page 1" ("Tab_Prueba04")) -> (error out=w963:errorcluster)  [unwired: 1 in, 1 out]
        n477 = property on="estado_ensayo_C" class="Str"(error in=w963, "Visible"=w965) -> (error out=w962:errorcluster)  [unwired: 1 in, 1 out]
        n478 = call "Queueu Comms Enqueue.vi"("error in"=w962, "Element"=T7 {"Estados"=enum."inicio", "Data"=variant}) -> ("error out"=w961:errorcluster)  [unwired: 8 in, 1 out]
        "ponderacion_C" <- w965
      }
      event "ir a inicio desde Z": Value Change {
        w972 = TRUE ("ponderacion_A")
        n479 = event-data() -> ()  [unwired: 1 in, 1 out]
        n480 = property on="Tab" class="TabCtl (strict)"(error in=w971, "Value"=T2."Page 1" ("Tab_Prueba04")) -> (error out=w970:errorcluster)  [unwired: 1 in, 1 out]
        n481 = property on="estado_ensayo_Z" class="Str"(error in=w970, "Visible"=w972) -> (error out=w969:errorcluster)  [unwired: 1 in, 1 out]
        n482 = call "Queueu Comms Enqueue.vi"("error in"=w969, "Element"=T7 {"Estados"=enum."inicio", "Data"=variant}) -> ("error out"=w968:errorcluster)  [unwired: 8 in, 1 out]
        "ponderacion_Z" <- w972
      }
      event "ir a resultados _Z": Value Change {
        n483 = event-data() -> ()  [unwired: 1 in, 1 out]
        n484 = property on="Tab" class="TabCtl (strict)"(error in=w977, "Value"=T2."Page 7" ("Tab_Prueba04")) -> (error out=w974:errorcluster)  [unwired: 1 in, 1 out]
        n485 = call "Queueu Comms Enqueue.vi"("error in"=w974, "Element"=T7 {"Estados"=enum."crea_voltajes_prueba_Z", "Data"=variant} ("Module Dat Cluster")) -> ("error out"=w975:errorcluster)  [unwired: 8 in, 1 out]
      }
      event "seguir": Value Change {
        n486 = event-data() -> ()  [unwired: 1 in, 1 out]
        n487 = local read "cumple_prueba04"() -> (w982:bool)
        n488 = call "Queueu Comms Enqueue.vi"("error in"=w979, "Element"=T7 {"Estados"=enum."salir", "Data"=variant}) -> ("error out"=w980:errorcluster)  [unwired: 8 in, 1 out]
        n489 = Select(t="Cumple", s=w982, f="No Cumple") -> (s? t:f=→"resultado":string)
      }
      event "Tabla_A": Value Change {
        n490 = event-data() -> ("NewVal"=w987:string[][])  [unwired: 1 in]
        n491 = Bundle By Name(cluster=T7 {"Estados"=enum."ingresaMedicionesA", "Data"=variant} ("Element"), "Estados"=Estados."ingresaMedicionesA", "Data"=w987) -> (w989:T7)
        n492 = call "Queueu Comms Enqueue.vi"("error in"=w992, "Element"=w989) -> ("error out"=w991:errorcluster)  [unwired: 8 in, 1 out]
      }
      event "Tabla_C": Value Change {
        n493 = event-data() -> ("NewVal"=w993:string[][])  [unwired: 1 in]
        n494 = Bundle By Name(cluster=T7 {"Estados"=enum."ingresaMedicionesA", "Data"=variant} ("Element"), "Estados"=Estados."ingresaMedicionesC", "Data"=w993) -> (w995:T7)
        n495 = call "Queueu Comms Enqueue.vi"("error in"=w998, "Element"=w995) -> ("error out"=w997:errorcluster)  [unwired: 8 in, 1 out]
      }
      event "Tabla_Z": Value Change {
        n496 = event-data() -> ("NewVal"=w999:string[][])  [unwired: 1 in]
        n497 = Bundle By Name(cluster=T7 {"Estados"=enum."ingresaMedicionesA", "Data"=variant} ("Element"), "Estados"=Estados."ingresaMedicionesZ", "Data"=w999) -> (w1001:T7)
        n498 = call "Queueu Comms Enqueue.vi"("error in"=w1004, "Element"=w1001) -> ("error out"=w1003:errorcluster)  [unwired: 8 in, 1 out]
      }
      event "cb_frec_A_2": Value Change {
        n499 = event-data() -> ("NewVal"=w1009:string)  [unwired: 1 in]
        n500 = property on="cb_frec_A_2" class="CmbBox"() -> ("Strings[]"=w1010:string[])  [unwired: 2 in, 2 out]
        n501 = Search 1D Array(1D array=w1010, element=w1009) -> (index of element=w1007:i32)  [unwired: 1 in]
        n502 = call "FGV_fila.vi"("error in (no error)"=w1006, "fila_inicial"=w1007, "action"=enum16{"increment", "set_start", "get"}."set_start") -> ("error out"=w1005:errorcluster)  [unwired: 1 in, 1 out]
        n503 = Bundle By Name(cluster=T7 {"Estados"=enum."iniciarGEN", "Data"=variant} ("Module Dat Cluster"), "Estados"=Estados."actualizarVrefA") -> (w1012:T7)
        n504 = call "Queueu Comms Enqueue.vi"("error in"=w1005, "Element"=w1012) -> ("error out"=w1011:errorcluster)  [unwired: 8 in, 1 out]
      }
      event "cb_frec_C_2": Value Change {
        n505 = event-data() -> ("NewVal"=w1020:string)  [unwired: 1 in]
        n506 = property on="cb_frec_C_2" class="CmbBox"() -> ("Strings[]"=w1015:string[])  [unwired: 2 in, 2 out]
        n507 = Search 1D Array(1D array=w1015, element=w1020) -> (index of element=w1018:i32)  [unwired: 1 in]
        n508 = call "FGV_fila.vi"("error in (no error)"=w1017, "fila_inicial"=w1018, "action"=enum16{"increment", "set_start", "get"}."set_start") -> ("error out"=w1016:errorcluster)  [unwired: 1 in, 1 out]
        n509 = Bundle By Name(cluster=T7 {"Estados"=enum."iniciarGEN", "Data"=variant} ("Module Dat Cluster"), "Estados"=Estados."actualizarVrefC") -> (w1022:T7)
        n510 = call "Queueu Comms Enqueue.vi"("error in"=w1016, "Element"=w1022) -> ("error out"=w1021:errorcluster)  [unwired: 8 in, 1 out]
      }
      event "cb_frec_Z_2": Value Change {
        n511 = event-data() -> ("NewVal"=w1030:string)  [unwired: 1 in]
        n512 = property on="cb_frec_Z_2" class="CmbBox"() -> ("Strings[]"=w1025:string[])  [unwired: 2 in, 2 out]
        n513 = Search 1D Array(1D array=w1025, element=w1030) -> (index of element=w1028:i32)  [unwired: 1 in]
        n514 = call "FGV_fila.vi"("error in (no error)"=w1027, "fila_inicial"=w1028, "action"=enum16{"increment", "set_start", "get"}."set_start") -> ("error out"=w1026:errorcluster)  [unwired: 1 in, 1 out]
        n515 = Bundle By Name(cluster=T7 {"Estados"=enum."iniciarGEN", "Data"=variant} ("Module Dat Cluster"), "Estados"=Estados."actualizarVrefZ") -> (w1032:T7)
        n516 = call "Queueu Comms Enqueue.vi"("error in"=w1026, "Element"=w1032) -> ("error out"=w1031:errorcluster)  [unwired: 8 in, 1 out]
      }
    }
  }
  n517 = disable-structure shown="Enabled" {
    frame Disabled {
      n518 = call "generar_frec.vi"() -> ()  [unwired: 10 in, 2 out]
      n519 = call "Queueu Comms Enqueue.vi"("Element"=T7 {"Estados"=enum."salir", "Data"=variant} ("Module Dat Cluster")) -> ()  [unwired: 9 in, 2 out]
    }
    frame Enabled {
    }
  }
  n520 = Merge Errors(w20, w19) -> (w17:errorcluster)
  n521 = call "Queue Cooms FGV.vi"("error in"=w17, "Action"=Queue_FGV_Action."Release") -> ("error out"=→"error out 2":errorcluster)  [unwired: 8 in, 1 out]
  "Prueba04 out" <- "Prueba04 in"
